vi "CRYGraph Window Menu.vi"(6 "MenuOption":string="View", 8 "pGraph VI":refnum<vi>, 9 "Flag Cluster":T1, 10 "Type":string="View", 11 "Runtime Menu Ref In":refnum<k9>) -> (3 "Runtime Menu Ref Out":refnum<k9>)   [LabVIEW 2013]
uses:
  Control/CRYFlag Cluster.ctl
  System.Windows.Forms
  CRYMainGlobal.vi
  CRYSystem/Task Sequence/CRYProject Run Control Global.vi
panel:
  in  "TextGraph":refnum<k24>(container)
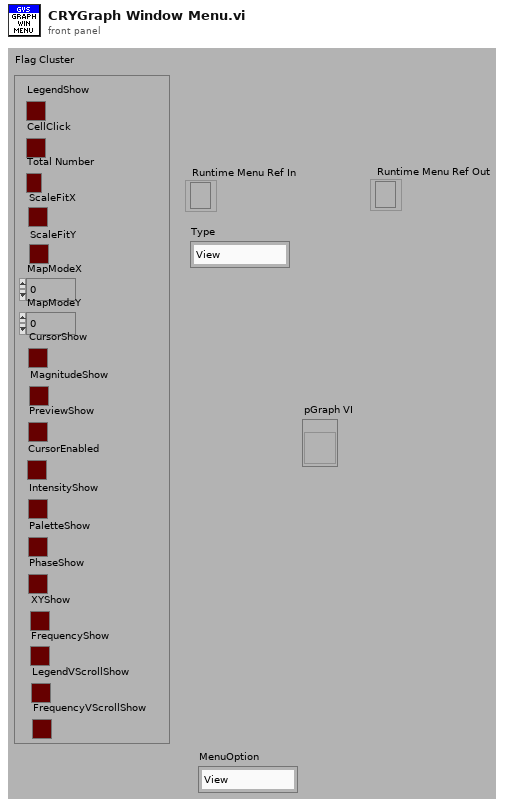
[diagram p1: front panel]
types:
  T1 = typedef "CRYFlag Cluster.ctl" = cluster{"LegendShow":bool, "CellClick":bool, "Total Number":bool, "ScaleFitX":bool, "ScaleFitY":bool, "MapModeX":u8, "MapModeY":u8, "CursorShow":bool, "MagnitudeShow":bool, "PreviewShow":bool, "CursorEnabled":bool, "IntensityShow":bool, "PaletteShow":bool, "PhaseShow":bool, "XYShow":bool, "FrequencyShow":bool, "LegendVScrollShow":bool, "FrequencyVScrollShow":bool}
  T2 = enum32{"English", "Chinese", "Korean", "Japanese", "Russian", "Chinese traditional"}
  T3 = typedef "LVRowAndColumnTypeDef.ctl" = cluster{"Row":i32, "Column":i32}
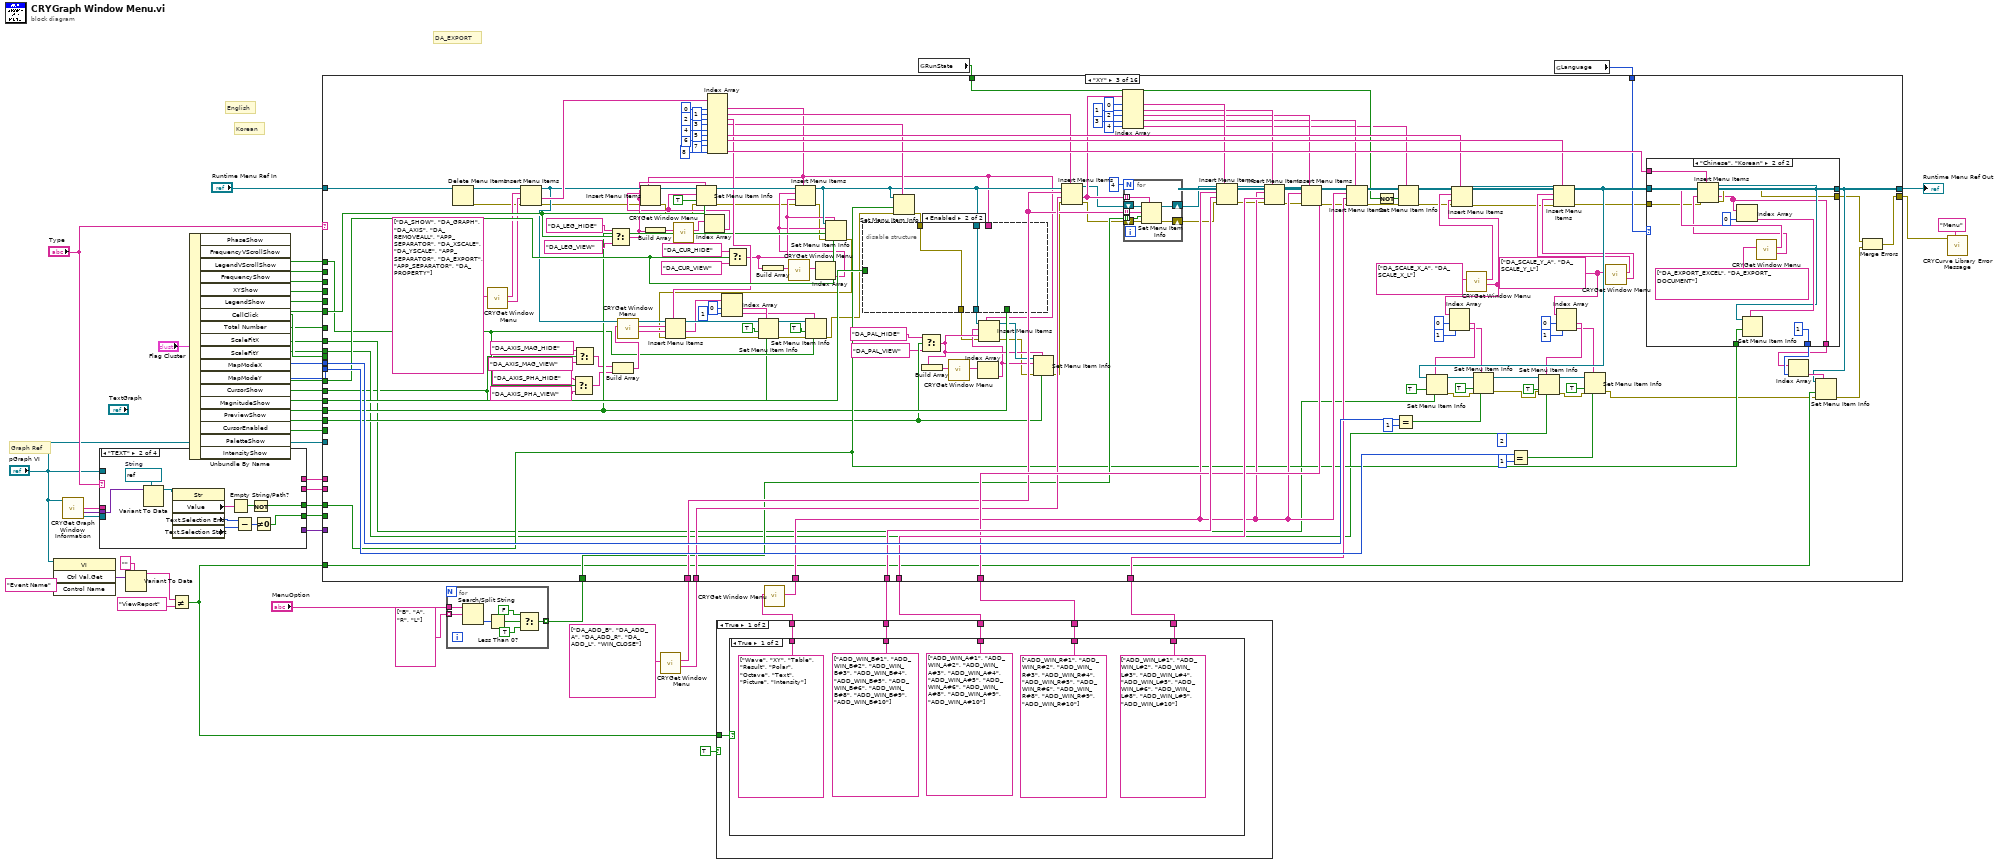
[diagram p0: block diagram]
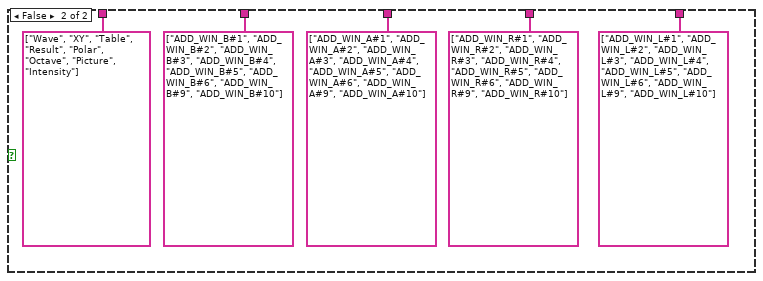
[diagram p2: hidden frame]
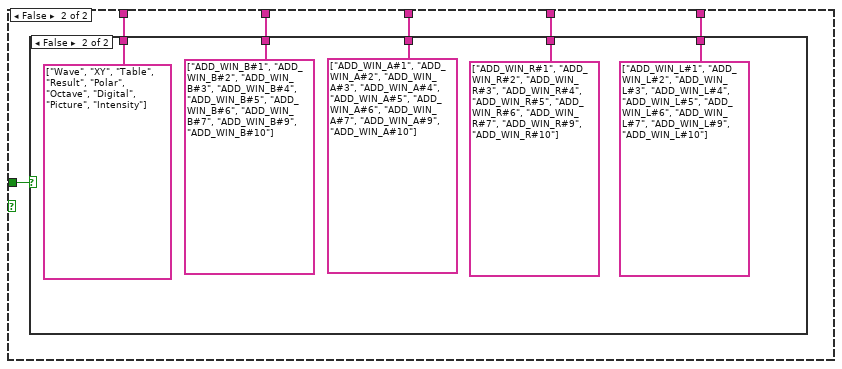
[diagram p3: hidden frame]
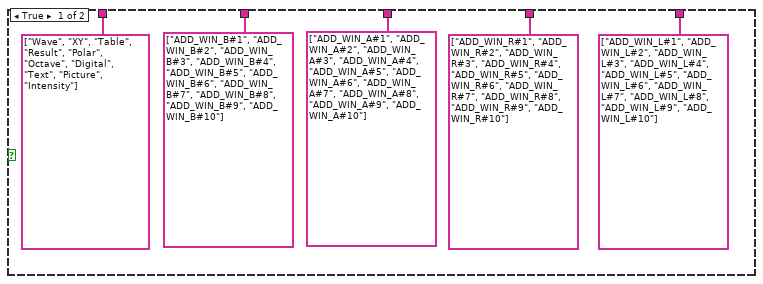
[diagram p4: hidden frame]
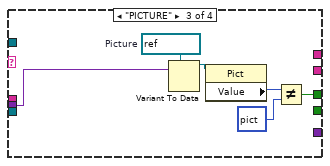
[diagram p6: hidden frame]
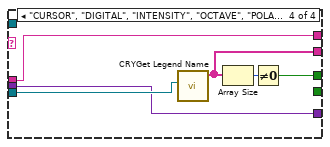
[diagram p7: hidden frame]
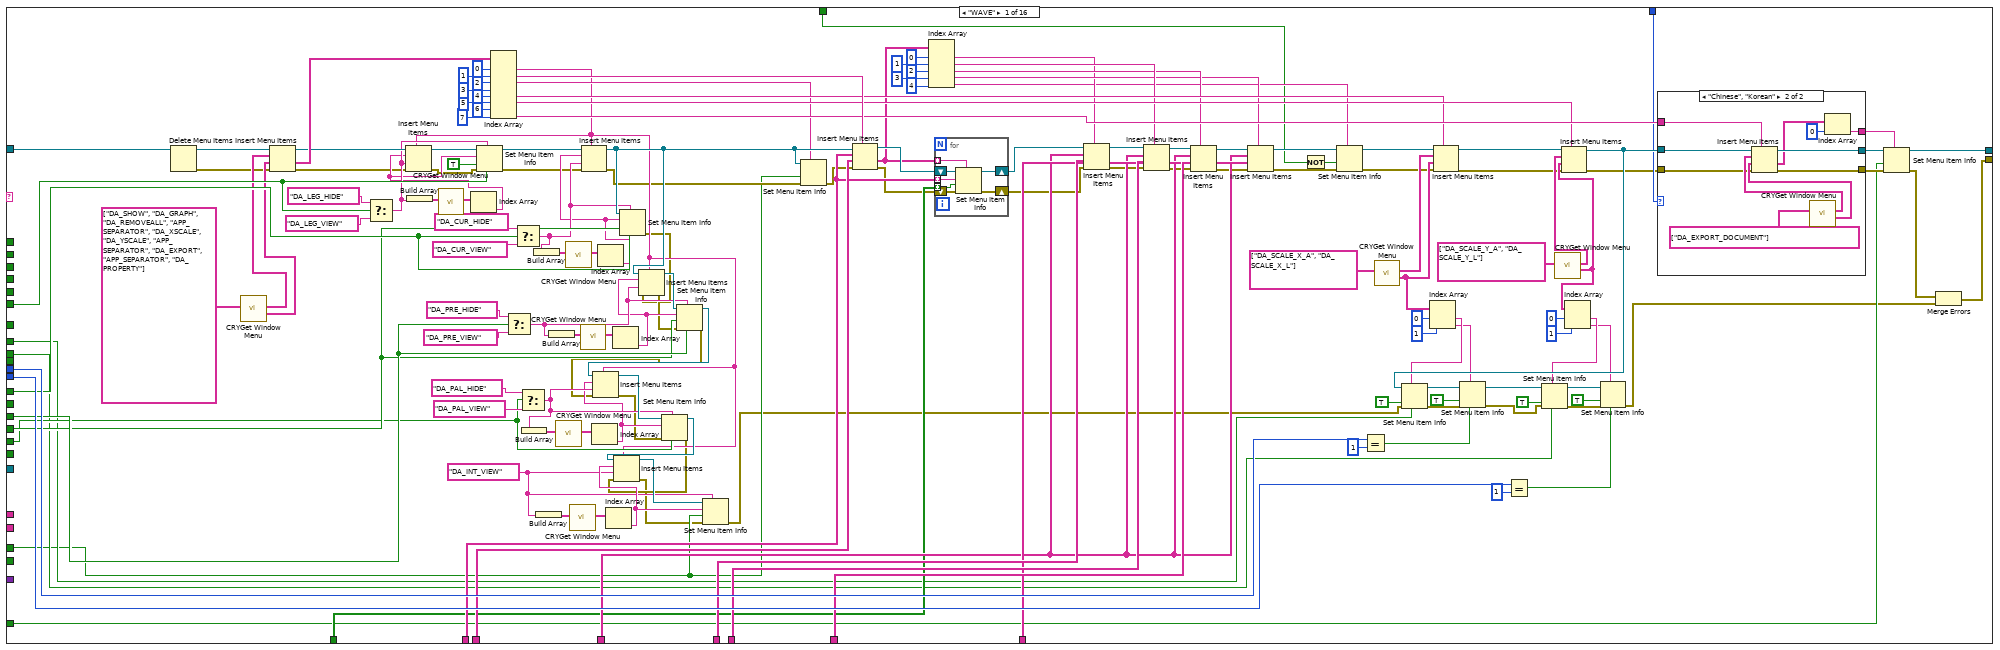
[diagram p8: hidden frame]
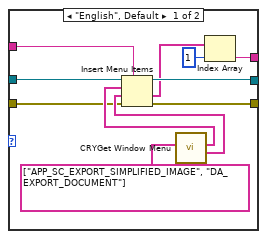
[diagram p9: hidden frame]
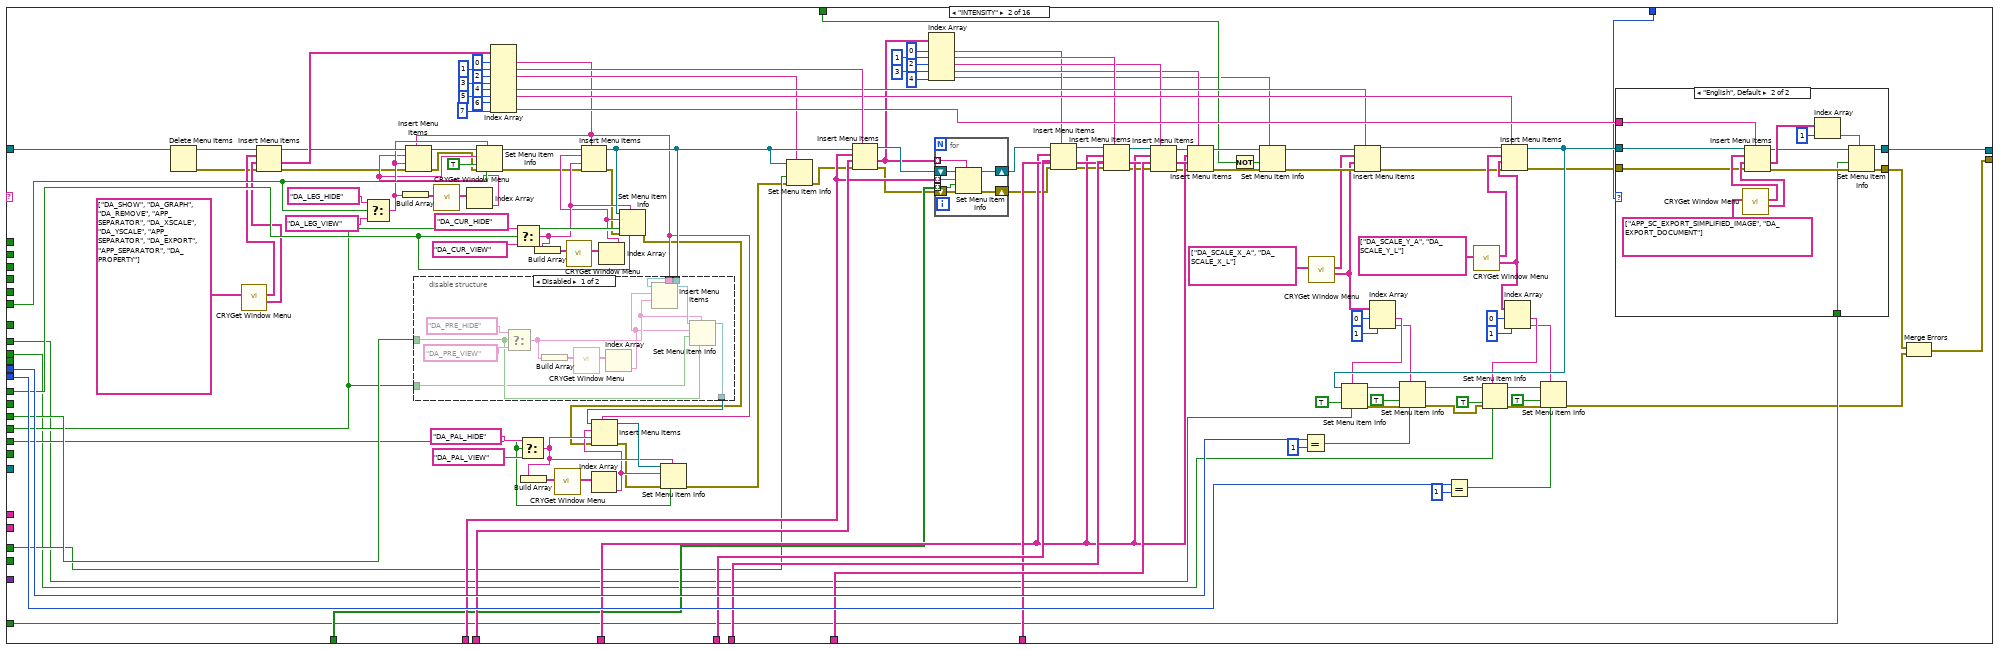
[diagram p10: hidden frame]
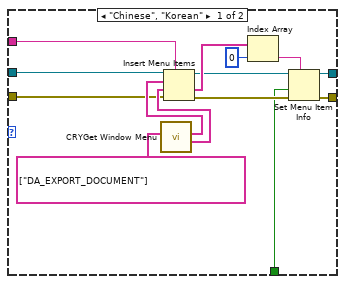
[diagram p11: hidden frame]
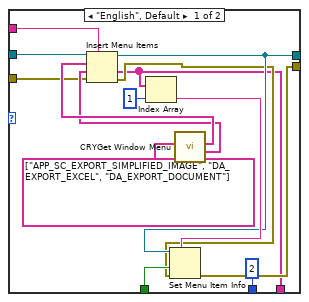
[diagram p13: hidden frame]
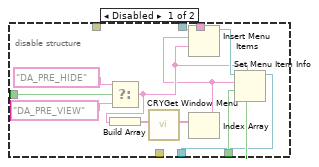
[diagram p14: hidden frame]
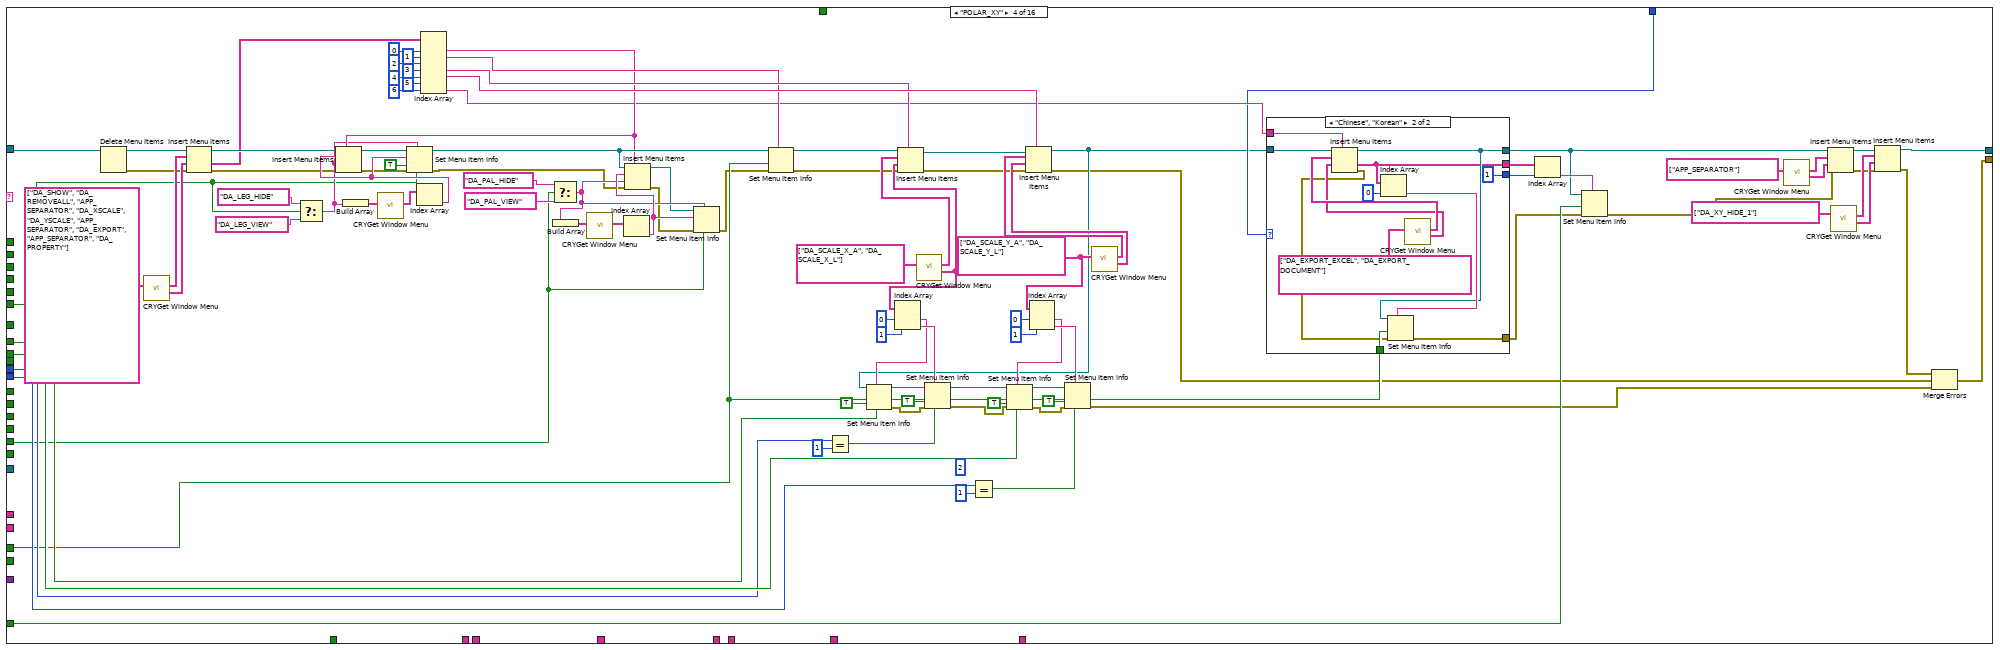
[diagram p15: hidden frame]
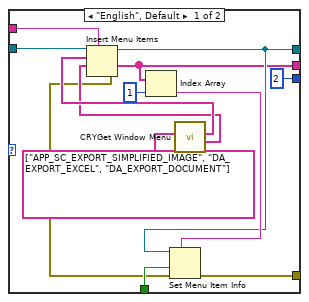
[diagram p16: hidden frame]
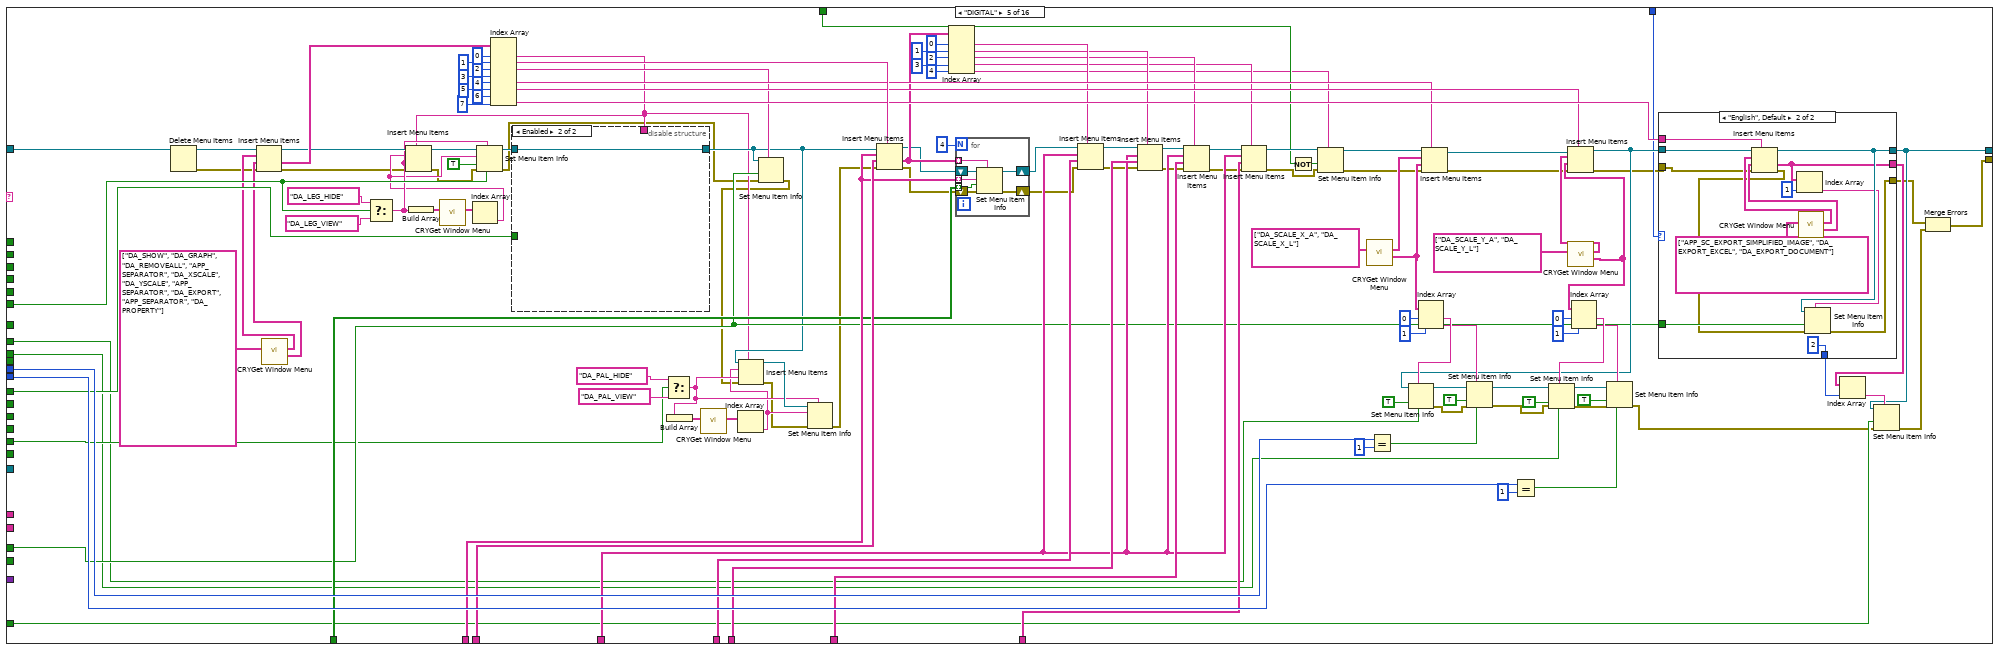
[diagram p17: hidden frame]
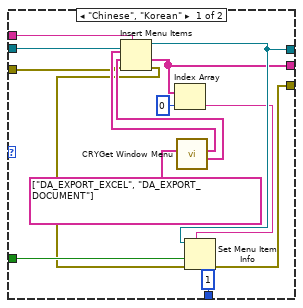
[diagram p18: hidden frame]
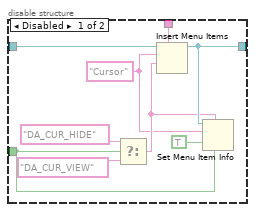
[diagram p19: hidden frame]
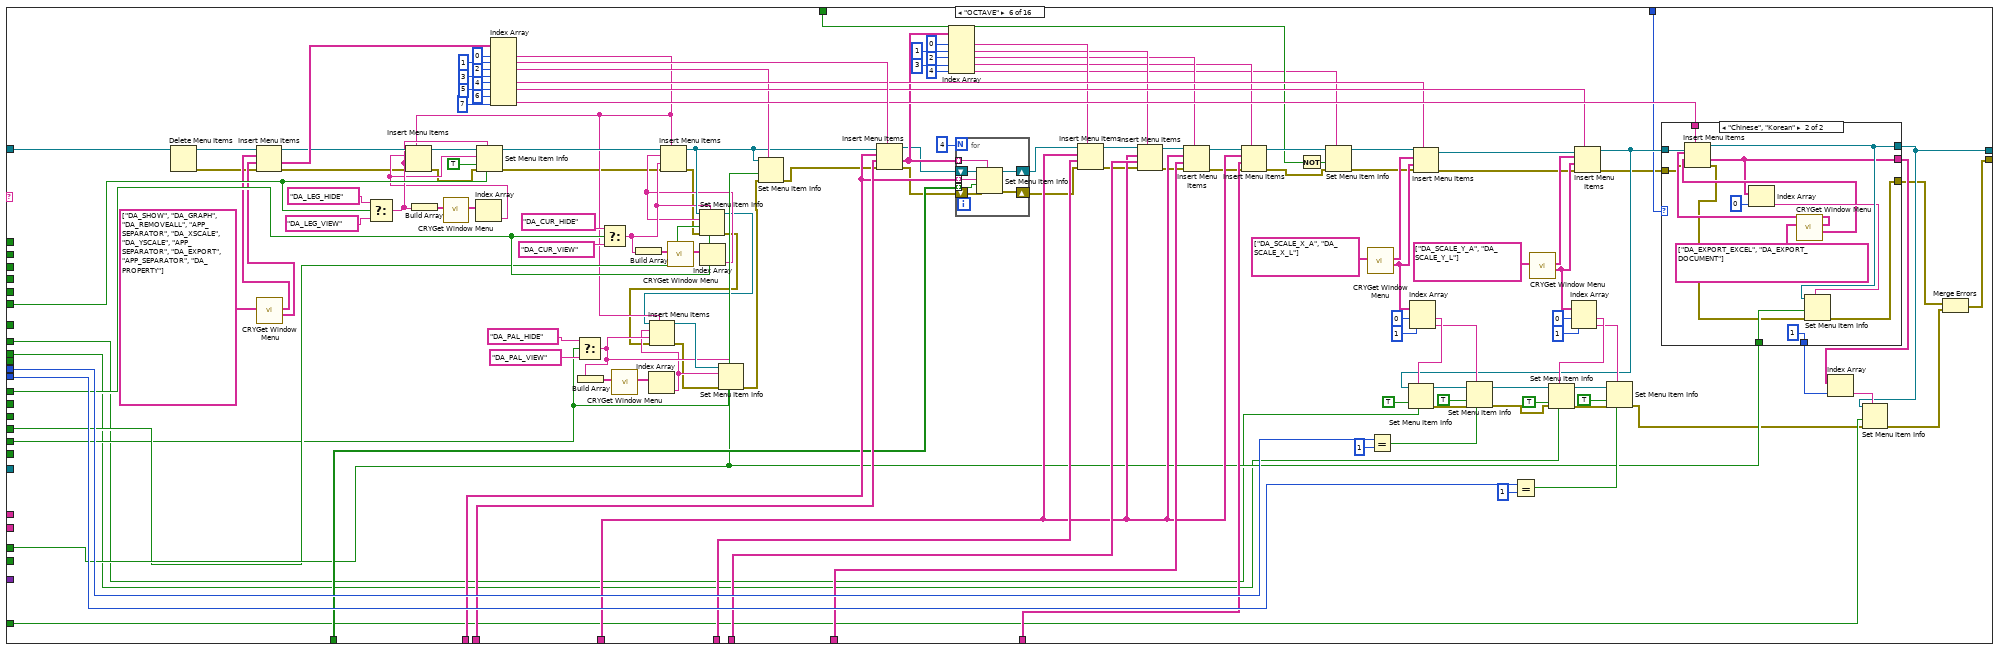
[diagram p20: hidden frame]
diagram:
  # "DA_EXPORT"
  # "Korean"
  # "English"
  # "Graph Ref"
  n1 = invoke class="VI" method="Ctrl Val.Get"(reference="pGraph VI", "Control Name"="Event Name") -> ("Get Control Value Variant"=w11:variant)  [unwired: 2 in, 3 out]
  n2 = call "CRYGet Graph Window Information.vi"("pGraph VI In"="pGraph VI") -> ("Graph Type Out"=w23:string, "Graph Control Ref Out"=w22:variant, "Legend Ref Out"=w21:refnum<vi>)  [unwired: 4 in, 8 out]
  n3 = case shown="\"TEXT\"" "Type" {
    tunnel: "pGraph VI" -> [_ _ _ _]
    tunnel: [_ w58 w67 w76] -> w35
    tunnel: [_ _ _ w75] -> w34
    tunnel: [w55 _ _ w74] -> w33
    tunnel: [_ _ _ w72] -> w32
    tunnel: [_ w57 _ _] -> w30
    tunnel: w23 -> [w55 _ _ w74]
    tunnel: w22 -> [_ w56 w66 w72]
    tunnel: w21 -> [_ _ _ w73]
    frame "INTENSITY_FLOAT", "LEGEND", Default {
    }
    frame "TEXT" {
      w59 = refnum<vi> refnum  # String
      n4 = Variant To Data(type=w59, Variant=w56) -> (data=w60:refnum<vi>)  [unwired: 1 in, 1 out]
      n5 = property class="Str"(reference=w60) -> ("Value"=w65:string, "Text.Selection End"=w61:u32, "Text.Selection Start"=w62:u32)  [unwired: 1 in, 2 out]
      n6 = Empty String/Path?(string/path=w65) -> (empty?=w64:bool)
      n7 = Subtract(x=w61, y=w62) -> (x-y=w63:u32)
      n8 = Not(x=w64) -> (.not. x?=w58:bool)
      n9 = Not Equal To 0?(x=w63) -> (x != 0?=w57:bool)
    }
    frame "PICTURE" {
      w71 = refnum<vi> refnum  # Picture
      n10 = Variant To Data(type=w71, Variant=w66) -> (data=w70:refnum<vi>)  [unwired: 1 in, 1 out]
      n11 = property class="Pict"(reference=w70) -> ("Value"=w69:picture)  [unwired: 1 in, 2 out]
      n12 = Not Equal?(x=w69, y=picture data[5B] ("Value")) -> (x != y?=w67:bool)
    }
    frame "CURSOR", "DIGITAL", "INTENSITY", "OCTAVE", "POLAR", "POLAR_XY", "PREVIEW", "RESULT", "TABLE", "WAVE", "XY" {
      n13 = call "CRYGet Legend Name.vi"("MCListbox Refnum"=w73) -> ("Names Out"=w75:string[])  [unwired: 10 in]
      n14 = Array Size(array=w75) -> (size(s)=w77:i32)
      n15 = Not Equal To 0?(x=w77) -> (x != 0?=w76:bool)
    }
  }
  n16 = Variant To Data(type="" ("Control Name"), Variant=w11) -> (data=w10:string)  [unwired: 1 in, 1 out]
  n17 = Not Equal?(x=w10, y="ViewReport" ("regular expression")) -> (x != y?=w6:bool)
  n18 = Unbundle By Name("Flag Cluster") -> ("PhaseShow"=w4:bool, "FrequencyVScrollShow"=w7:bool, "LegendVScrollShow"=w8:bool, "FrequencyShow"=w16:bool, "XYShow"=w17:bool, "LegendShow"=w52:bool, "CellClick"=w42:bool, "Total Number"=w43:bool, "ScaleFitX"=w19:bool, "ScaleFitY"=w20:bool, "MapModeX"=w50:u8, "MapModeY"=w49:u8, "CursorShow"=w44:bool, "MagnitudeShow"=w41:bool, "PreviewShow"=w40:bool, "CursorEnabled"=w39:bool, "PaletteShow"=w25:bool, "IntensityShow"=w24:bool)
  n19 = for {
    tunnel: "MenuOption" -> [w84]
    tunnel: string[] ["B", "A", "R", "L"] -> [w83] mode=indexing
    tunnel: [w78] -> w37 mode=indexing
    n20 = Search/Split String(string=w84, search string/char (-)=w83) -> (offset of match=w82:i32)  [unwired: 1 in, 2 out]
    n21 = Less Than 0?(x=w82) -> (x < 0?=w81:bool)
    n22 = Select(t=FALSE ("enabled"), s=w81, f=TRUE ("enabled")) -> (s? t:f=w78:bool)
  }
  n23 = call "CRYGet Window Menu.vi"("Tags"=string[] ["DA_ADD_B", "DA_ADD_A", "DA_ADD_R", "DA_ADD_L", "WIN_CLOSE"]) -> ("Tags_Out"=w27:string[], "Names_Out"=w28:string[])  [unwired: 8 in, 1 out]
  n24 = case shown="True" TRUE {
    tunnel: [w90 w106] -> w48
    tunnel: [w89 w105] -> w47
    tunnel: [w88 w104] -> w46
    tunnel: [w87 w103] -> w45
    tunnel: w6 -> [w86 w102]
    tunnel: [w85 w101] -> w5
    frame True {
      n25 = case shown="True" w86 {
        tunnel: [string[] ["ADD_WIN_L#1", "ADD_WIN_L#2", "ADD_WIN_L#3", "ADD_WIN_L#4", "ADD_WIN_L#5", "ADD_WIN_L#6", "ADD_WIN_L#8", "ADD_WIN_L#9", "ADD_WIN_L#10"] string[] ["ADD_WIN_L#1", "ADD_WIN_L#2", "ADD_WIN_L#3", "ADD_WIN_L#4", "ADD_WIN_L#5", "ADD_WIN_L#6", "ADD_WIN_L#9", "ADD_WIN_L#10"]] -> w90
        tunnel: [string[] ["ADD_WIN_R#1", "ADD_WIN_R#2", "ADD_WIN_R#3", "ADD_WIN_R#4", "ADD_WIN_R#5", "ADD_WIN_R#6", "ADD_WIN_R#8", "ADD_WIN_R#9", "ADD_WIN_R#10"] string[] ["ADD_WIN_R#1", "ADD_WIN_R#2", "ADD_WIN_R#3", "ADD_WIN_R#4", "ADD_WIN_R#5", "ADD_WIN_R#6", "ADD_WIN_R#9", "ADD_WIN_R#10"]] -> w89
        tunnel: [string[] ["ADD_WIN_B#1", "ADD_WIN_B#2", "ADD_WIN_B#3", "ADD_WIN_B#4", "ADD_WIN_B#5", "ADD_WIN_B#6", "ADD_WIN_B#8", "ADD_WIN_B#9", "ADD_WIN_B#10"] string[] ["ADD_WIN_B#1", "ADD_WIN_B#2", "ADD_WIN_B#3", "ADD_WIN_B#4", "ADD_WIN_B#5", "ADD_WIN_B#6", "ADD_WIN_B#9", "ADD_WIN_B#10"]] -> w88
        tunnel: [string[] ["ADD_WIN_A#1", "ADD_WIN_A#2", "ADD_WIN_A#3", "ADD_WIN_A#4", "ADD_WIN_A#5", "ADD_WIN_A#6", "ADD_WIN_A#8", "ADD_WIN_A#9", "ADD_WIN_A#10"] string[] ["ADD_WIN_A#1", "ADD_WIN_A#2", "ADD_WIN_A#3", "ADD_WIN_A#4", "ADD_WIN_A#5", "ADD_WIN_A#6", "ADD_WIN_A#9", "ADD_WIN_A#10"]] -> w87
        tunnel: [string[] ["Wave", "XY", "Table", "Result", "Polar", "Octave", "Text", "Picture", "Intensity"] string[] ["Wave", "XY", "Table", "Result", "Polar", "Octave", "Picture", "Intensity"]] -> w85
        frame True {
        }
        frame False {
        }
      }
    }
    frame False {
      n26 = case shown="False" w102 {
        tunnel: [string[] ["ADD_WIN_L#1", "ADD_WIN_L#2", "ADD_WIN_L#3", "ADD_WIN_L#4", "ADD_WIN_L#5", "ADD_WIN_L#6", "ADD_WIN_L#7", "ADD_WIN_L#8", "ADD_WIN_L#9", "ADD_WIN_L#10"] string[] ["ADD_WIN_L#1", "ADD_WIN_L#2", "ADD_WIN_L#3", "ADD_WIN_L#4", "ADD_WIN_L#5", "ADD_WIN_L#6", "ADD_WIN_L#7", "ADD_WIN_L#9", "ADD_WIN_L#10"]] -> w106
        tunnel: [string[] ["ADD_WIN_R#1", "ADD_WIN_R#2", "ADD_WIN_R#3", "ADD_WIN_R#4", "ADD_WIN_R#5", "ADD_WIN_R#6", "ADD_WIN_R#7", "ADD_WIN_R#8", "ADD_WIN_R#9", "ADD_WIN_R#10"] string[] ["ADD_WIN_R#1", "ADD_WIN_R#2", "ADD_WIN_R#3", "ADD_WIN_R#4", "ADD_WIN_R#5", "ADD_WIN_R#6", "ADD_WIN_R#7", "ADD_WIN_R#9", "ADD_WIN_R#10"]] -> w105
        tunnel: [string[] ["ADD_WIN_B#1", "ADD_WIN_B#2", "ADD_WIN_B#3", "ADD_WIN_B#4", "ADD_WIN_B#5", "ADD_WIN_B#6", "ADD_WIN_B#7", "ADD_WIN_B#8", "ADD_WIN_B#9", "ADD_WIN_B#10"] string[] ["ADD_WIN_B#1", "ADD_WIN_B#2", "ADD_WIN_B#3", "ADD_WIN_B#4", "ADD_WIN_B#5", "ADD_WIN_B#6", "ADD_WIN_B#7", "ADD_WIN_B#9", "ADD_WIN_B#10"]] -> w104
        tunnel: [string[] ["ADD_WIN_A#1", "ADD_WIN_A#2", "ADD_WIN_A#3", "ADD_WIN_A#4", "ADD_WIN_A#5", "ADD_WIN_A#6", "ADD_WIN_A#7", "ADD_WIN_A#8", "ADD_WIN_A#9", "ADD_WIN_A#10"] string[] ["ADD_WIN_A#1", "ADD_WIN_A#2", "ADD_WIN_A#3", "ADD_WIN_A#4", "ADD_WIN_A#5", "ADD_WIN_A#6", "ADD_WIN_A#7", "ADD_WIN_A#9", "ADD_WIN_A#10"]] -> w103
        tunnel: [string[] ["Wave", "XY", "Table", "Result", "Polar", "Octave", "Digital", "Text", "Picture", "Intensity"] string[] ["Wave", "XY", "Table", "Result", "Polar", "Octave", "Digital", "Picture", "Intensity"]] -> w101
        frame True {
        }
        frame False {
        }
      }
    }
  }
  n27 = call "CRYGet Window Menu.vi"("Tags"=w5) -> ("Names_Out"=w26:string[])  [unwired: 8 in, 2 out]
  n28 = global read "CRYProject Run Control Global.vi" "RunState"() -> (w15:bool)
  n29 = global read "CRYMainGlobal.vi" "Language"() -> (w18:T2)
  n30 = case shown="\"XY\"" "Type" {
    tunnel: "Runtime Menu Ref In" -> [w269 w435 w644 w736 w950 w1136 w1273 w1372 w1457 w1527 w1600 w1619 w1701 w1737 w1832 w1835]
    tunnel: w52 -> [w222 w409 w596 w735 w902 w1088 _ _ _ _ _ _ _ _ _ _]
    tunnel: w43 -> [_ _ _ _ _ _ _ _ _ _ _ w1615 w1698 _ _ _]
    tunnel: [w133 w309 w509 w729 w838 w1014 w1184 w1294 w1384 w1469 w1537 w1620 w1702 w1735 w1830 w1834] -> w53
    tunnel: w50 -> [w242 w427 w617 w732 w923 w1109 _ _ _ _ _ _ _ _ _ _]
    tunnel: w49 -> [w240 w426 w615 w731 w921 w1107 _ _ _ _ _ _ _ _ _ _]
    tunnel: w42 -> [_ _ _ _ _ _ _ _ _ _ _ w1616 w1699 _ _ _]
    tunnel: w19 -> [w166 w371 w543 w734 w866 w1044 _ _ _ _ _ _ _ _ _ _]
    tunnel: w20 -> [w165 w370 w542 w733 w865 w1043 _ _ _ _ _ _ _ _ _ _]
    tunnel: w48 -> [w225 w412 w599 _ w905 w1091 w1255 w1364 w1449 w1520 w1594 _ _ _ _ _]
    tunnel: w47 -> [w226 w413 w600 _ w906 w1092 w1256 w1363 w1448 w1519 w1593 _ _ _ _ _]
    tunnel: w46 -> [w228 w415 w602 _ w908 w1094 w1258 w1362 w1447 w1518 w1592 _ _ _ _ _]
    tunnel: w45 -> [w227 w414 w601 _ w907 w1093 w1257 w1361 w1446 w1517 w1591 _ _ _ _ _]
    tunnel: w28 -> [w209 w399 w579 _ w896 w1082 w1246 w1347 w1432 w1504 w1578 _ _ _ _ _]
    tunnel: w27 -> [w223 w410 w597 _ w903 w1089 w1253 w1360 w1445 w1516 w1590 _ _ _ _ _]
    tunnel: w26 -> [w224 w411 w598 _ w904 w1090 w1254 w1359 w1444 w1515 w1589 _ _ _ _ _]
    tunnel: w44 -> [w217 w404 w591 _ w899 w1085 _ _ _ _ _ _ _ w1734 _ _]
    tunnel: w41 -> [_ _ w492 _ _ _ _ _ _ _ _ _ _ _ _ _]
    tunnel: w40 -> [w213 w403 w576 _ _ _ _ _ _ _ _ _ _ _ _ _]
    tunnel: w39 -> [w206 w396 w574 _ _ w1072 _ _ _ _ _ _ _ _ _ _]
    tunnel: w37 -> [w208 w398 w578 _ w895 w1081 w1245 w1346 w1431 w1503 w1577 _ _ _ _ _]
    tunnel: w35 -> [w149 w393 w575 w726 w890 w1075 w1189 w1298 w1414 w1499 w1567 _ _ _ _ _]
    tunnel: w34 -> [_ _ _ _ _ _ _ _ _ _ _ _ _ w1730 _ _]
    tunnel: w33 -> [_ _ _ _ _ _ _ _ _ _ _ w1609 w1697 w1725 _ _]
    tunnel: w32 -> [_ _ _ _ _ _ _ w1328 _ _ _ _ _ w1729 _ _]
    tunnel: w30 -> [_ _ _ _ _ _ _ _ _ _ w1566 _ _ _ _ _]
    tunnel: w25 -> [w175 w372 w546 w730 w867 w1047 _ _ _ _ _ _ _ _ _ _]
    tunnel: w24 -> [_ _ _ _ _ _ _ _ _ _ _ _ _ _ _ _]
    tunnel: "pGraph VI" -> [_ _ _ _ _ _ _ _ w1418 _ _ _ _ _ _ _]
    tunnel: w18 -> [w164 w307 w541 w727 w864 w1042 _ _ _ _ _ _ _ _ _ _]
    tunnel: [w117 w302 w489 w702 w830 w1006 w1183 w1292 w1382 w1467 w1536 w1611 w1676 w1721 w1825 w1833] -> w2
    tunnel: w17 -> [_ _ _ _ _ _ w1215 _ _ _ _ _ _ _ _ _]
    tunnel: w16 -> [_ _ _ _ _ _ w1214 _ _ _ _ _ _ _ _ _]
    tunnel: w15 -> [w144 w349 w515 _ w842 w1020 w1200 w1307 w1397 w1484 w1543 _ _ _ _ _]
    tunnel: w6 -> [w130 w308 w508 w720 w835 w1011 w1182 w1291 w1381 w1466 _ _ _ _ _ _]
    tunnel: w8 -> [_ _ _ _ _ _ _ _ _ _ _ w1610 _ _ _ _]
    tunnel: w7 -> [_ _ _ _ _ _ _ _ _ _ _ _ w1675 _ _ _]
    tunnel: w4 -> [_ _ w493 _ _ _ _ _ _ _ _ _ _ _ _ _]
    frame "WAVE" {
      w167 = "DA_INT_VIEW"
      n31 = Delete Menu Items(9:w269) -> (0:w163:errorcluster, 3:w272:refnum<k9>)  [unwired: 1 in, 2 out]
      n32 = call "CRYGet Window Menu.vi"("Tags"=string[] ["DA_SHOW", "DA_GRAPH", "DA_REMOVEALL", "APP_SEPARATOR", "DA_XSCALE", "DA_YSCALE", "APP_SEPARATOR", "DA_EXPORT", "APP_SEPARATOR", "DA_PROPERTY"]) -> ("Tags_Out"=w201:string[], "Names_Out"=w202:string[])  [unwired: 8 in, 1 out]
      n33 = Insert Menu Items(6:w163, 7:w201, 8:w202, 9:w272) -> (0:w162:errorcluster, 1:w271:string[], 3:w268:refnum<k9>)  [unwired: 2 out]
      n34 = Select(t="DA_LEG_HIDE", s=w222, f="DA_LEG_VIEW") -> (s? t:f=w198:string)
      n35 = Build Array(w198) -> (w200:string[])
      n36 = call "CRYGet Window Menu.vi"("Tags"=w200) -> ("Names_Out"=w199:string[])  [unwired: 8 in, 2 out]
      n37 = Index Array(array=w199) -> (element=w197:string)  [unwired: 1 in]
      n38 = Index Array(array=w271, index #1=0 ("index"), index #2=1 ("index"), index #3=2 ("index"), index #4=3 ("index"), index #5=4 ("index"), index #6=5 ("index"), index #7=6 ("index"), index #8=7 ("index")) -> (element #1=w169:string, element #2=w270:string, element #3=w204:string, element #5=w253:string, element #6=w254:string, element #8=w264:string)  [unwired: 2 out]
      n39 = Insert Menu Items(5:w169, 6:w162, 7:w198, 8:w197, 9:w268) -> (0:w161:errorcluster, 3:w267:refnum<k9>)  [unwired: 1 in, 1 out]
      n40 = Set Menu Item Info(6:w222, 7:w198, 8:w161, 9:TRUE ("enabled"), 10:w197, 11:w267) -> (0:w160:errorcluster, 3:w266:refnum<k9>)  [unwired: 1 out]
      n41 = Select(t="DA_PRE_HIDE", s=w213, f="DA_PRE_VIEW") -> (s? t:f=w184:string)
      n42 = Select(t="DA_CUR_HIDE", s=w217, f="DA_CUR_VIEW") -> (s? t:f=w194:string)
      n43 = Select(t="DA_PAL_HIDE", s=w175, f="DA_PAL_VIEW") -> (s? t:f=w179:string)
      n44 = Build Array(w179) -> (w182:string[])
      n45 = Build Array(w194) -> (w196:string[])
      n46 = Build Array(w167) -> (w172:string[])
      n47 = Build Array(w184) -> (w185:string[])
      n48 = call "CRYGet Window Menu.vi"("Tags"=w182) -> ("Names_Out"=w181:string[])  [unwired: 8 in, 2 out]
      n49 = call "CRYGet Window Menu.vi"("Tags"=w196) -> ("Names_Out"=w195:string[])  [unwired: 8 in, 2 out]
      n50 = call "CRYGet Window Menu.vi"("Tags"=w172) -> ("Names_Out"=w173:string[])  [unwired: 8 in, 2 out]
      n51 = call "CRYGet Window Menu.vi"("Tags"=w185) -> ("Names_Out"=w186:string[])  [unwired: 8 in, 2 out]
      n52 = Index Array(array=w181) -> (element=w178:string)  [unwired: 1 in]
      n53 = Index Array(array=w195) -> (element=w193:string)  [unwired: 1 in]
      n54 = Insert Menu Items(5:w169, 6:w160, 7:w194, 8:w193, 9:w266) -> (0:w159:errorcluster, 3:w205:refnum<k9>)  [unwired: 2 out]
      n55 = Index Array(array=w173) -> (element=w168:string)  [unwired: 1 in]
      n56 = Index Array(array=w186) -> (element=w183:string)  [unwired: 1 in]
      n57 = Set Menu Item Info(6:w217, 7:w194, 9:w206, 10:w193, 11:w205) -> (0:w124:errorcluster)  [unwired: 1 in, 2 out]
      n58 = Insert Menu Items(5:w169, 6:w124, 7:w184, 8:w183, 9:w205) -> (0:w129:errorcluster, 3:w214:refnum<k9>)  [unwired: 2 out]
      n59 = Set Menu Item Info(6:w213, 7:w184, 8:w129, 9:w206, 10:w183, 11:w214) -> (0:w128:errorcluster, 3:w174:refnum<k9>)  [unwired: 1 out]
      n60 = Insert Menu Items(5:w169, 6:w128, 7:w179, 8:w178, 9:w174) -> (0:w127:errorcluster, 3:w180:refnum<k9>)  [unwired: 2 out]
      n61 = Set Menu Item Info(6:w175, 7:w179, 8:w127, 10:w178, 11:w180) -> (0:w126:errorcluster, 3:w171:refnum<k9>)  [unwired: 1 in, 1 out]
      n62 = Insert Menu Items(5:w169, 6:w126, 7:w167, 8:w168, 9:w171) -> (0:w125:errorcluster, 3:w170:refnum<k9>)  [unwired: 2 out]
      n63 = Set Menu Item Info(7:w167, 8:w125, 9:w149, 10:w168, 11:w170) -> (0:w123:errorcluster)  [unwired: 1 in, 2 out]
      n64 = Set Menu Item Info(7:w204, 8:w159, 9:w149, 11:w205) -> (0:w158:errorcluster)  [unwired: 1 in, 3 out]
      n65 = Insert Menu Items(5:w270, 6:w158, 7:w223, 8:w209, 9:w205) -> (0:w157:errorcluster, 1:w210:string[], 3:w211:refnum<k9>)  [unwired: 1 out]
      n66 = Index Array(array=w210, index #1=0 ("index"), index #2=1 ("index"), index #3=2 ("index"), index #4=3 ("index"), index #5=4 ("index")) -> (element #1=w212:string, element #2=w234:string, element #3=w233:string, element #4=w232:string, element #5=w145:string)
      n67 = for {
        tunnel: w210 -> [w300] mode=indexing
        tunnel: w209 -> [w299] mode=indexing
        tunnel: w208 -> [w298] mode=indexing
        shift-right: [w297] -> w207
        shift-left: w211 -> [w301]
        shift-right: [w295] -> w156
        shift-left: w157 -> [w296]
        n68 = Set Menu Item Info(7:w300, 8:w296, 9:w298, 10:w299, 11:w301) -> (0:w295:errorcluster, 3:w297:refnum<k9>)  [unwired: 1 in, 1 out]
      }
      n69 = Insert Menu Items(5:w212, 6:w156, 7:w228, 8:w224, 9:w207) -> (0:w155:errorcluster, 3:w231:refnum<k9>)  [unwired: 2 out]
      n70 = Insert Menu Items(5:w234, 6:w155, 7:w227, 8:w224, 9:w231) -> (0:w154:errorcluster, 3:w230:refnum<k9>)  [unwired: 2 out]
      n71 = Insert Menu Items(5:w233, 6:w154, 7:w226, 8:w224, 9:w230) -> (0:w153:errorcluster, 3:w229:refnum<k9>)  [unwired: 2 out]
      n72 = Insert Menu Items(5:w232, 6:w153, 7:w225, 8:w224, 9:w229) -> (0:w152:errorcluster, 3:w147:refnum<k9>)  [unwired: 2 out]
      n73 = Not(x=w144) -> (.not. x?=w143:bool)
      n74 = Set Menu Item Info(7:w145, 9:w143, 11:w147) -> (3:w146:refnum<k9>)  [unwired: 2 in, 3 out]
      n75 = Equal?(x=w242, y=u8 1) -> (x = y?=w241:bool)
      n76 = call "CRYGet Window Menu.vi"("Tags"=string[] ["DA_SCALE_X_A", "DA_SCALE_X_L"]) -> ("Tags_Out"=w190:string[], "Names_Out"=w191:string[])  [unwired: 8 in, 1 out]
      n77 = Index Array(array=w190, index #1=0 ("index"), index #2=1 ("index")) -> (element #1=w250:string, element #2=w249:string)
      n78 = Insert Menu Items(5:w253, 6:w152, 7:w190, 8:w191, 9:w146) -> (0:w151:errorcluster, 3:w263:refnum<k9>)  [unwired: 2 out]
      n79 = Equal?(x=w240, y=u8 1) -> (x = y?=w239:bool)
      n80 = call "CRYGet Window Menu.vi"("Tags"=string[] ["DA_SCALE_Y_A", "DA_SCALE_Y_L"]) -> ("Tags_Out"=w187:string[], "Names_Out"=w188:string[])  [unwired: 8 in, 1 out]
      n81 = Insert Menu Items(5:w254, 6:w151, 7:w187, 8:w188, 9:w263) -> (0:w150:errorcluster, 3:w261:refnum<k9>)  [unwired: 2 out]
      n82 = Set Menu Item Info(6:w166, 7:w250, 8:w123, 9:TRUE ("enabled"), 11:w261) -> (0:w122:errorcluster, 3:w260:refnum<k9>)  [unwired: 2 out]
      n83 = Set Menu Item Info(6:w241, 7:w249, 8:w122, 9:TRUE ("enabled"), 11:w260) -> (0:w121:errorcluster, 3:w256:refnum<k9>)  [unwired: 2 out]
      n84 = Index Array(array=w187, index #1=0 ("index"), index #2=1 ("index")) -> (element #1=w246:string, element #2=w245:string)
      n85 = Set Menu Item Info(6:w165, 7:w246, 8:w121, 9:TRUE ("enabled"), 11:w256) -> (0:w120:errorcluster, 3:w255:refnum<k9>)  [unwired: 2 out]
      n86 = Set Menu Item Info(6:w239, 7:w245, 8:w120, 9:TRUE ("enabled"), 11:w255) -> (0:w118:errorcluster)  [unwired: 3 out]
      n87 = case shown="\"Chinese\", \"Korean\"" w164 {
        tunnel: w264 -> [w283 w294]
        tunnel: w261 -> [w282 w293]
        tunnel: [w281 w292] -> w134
        tunnel: w150 -> [w278 w289]
        tunnel: [w277 w288] -> w132
        tunnel: [w273 w284] -> w131
        frame "English", Default {
          n88 = call "CRYGet Window Menu.vi"("Tags"=string[] ["APP_SC_EXPORT_SIMPLIFIED_IMAGE", "DA_EXPORT_DOCUMENT"]) -> ("Tags_Out"=w279:string[], "Names_Out"=w280:string[])  [unwired: 8 in, 1 out]
          n89 = Insert Menu Items(5:w283, 6:w278, 7:w279, 8:w280, 9:w282) -> (0:w277:errorcluster, 1:w274:string[], 3:w281:refnum<k9>)  [unwired: 1 out]
          n90 = Index Array(array=w274, index=1) -> (element=w273:string)
        }
        frame "Chinese", "Korean" {
          n91 = call "CRYGet Window Menu.vi"("Tags"=string[] ["DA_EXPORT_DOCUMENT"]) -> ("Tags_Out"=w290:string[], "Names_Out"=w291:string[])  [unwired: 8 in, 1 out]
          n92 = Insert Menu Items(5:w294, 6:w289, 7:w290, 8:w291, 9:w293) -> (0:w288:errorcluster, 1:w285:string[], 3:w292:refnum<k9>)  [unwired: 1 out]
          n93 = Index Array(array=w285, index=0) -> (element=w284:string)
        }
      }
      n94 = Set Menu Item Info(7:w131, 8:w132, 9:w130, 11:w134) -> (0:w119:errorcluster, 3:w133:refnum<k9>)  [unwired: 2 in, 1 out]
      n95 = Merge Errors(w119, w118) -> (w117:errorcluster)
    }
    frame "INTENSITY" {
      n96 = Delete Menu Items(9:w435) -> (0:w369:errorcluster, 3:w438:refnum<k9>)  [unwired: 1 in, 2 out]
      n97 = call "CRYGet Window Menu.vi"("Tags"=string[] ["DA_SHOW", "DA_GRAPH", "DA_REMOVE", "APP_SEPARATOR", "DA_XSCALE", "DA_YSCALE", "APP_SEPARATOR", "DA_EXPORT", "APP_SEPARATOR", "DA_PROPERTY"]) -> ("Tags_Out"=w390:string[], "Names_Out"=w391:string[])  [unwired: 8 in, 1 out]
      n98 = Insert Menu Items(6:w369, 7:w390, 8:w391, 9:w438) -> (0:w368:errorcluster, 1:w437:string[], 3:w434:refnum<k9>)  [unwired: 2 out]
      n99 = Select(t="DA_LEG_HIDE", s=w409, f="DA_LEG_VIEW") -> (s? t:f=w387:string)
      n100 = Build Array(w387) -> (w389:string[])
      n101 = call "CRYGet Window Menu.vi"("Tags"=w389) -> ("Names_Out"=w388:string[])  [unwired: 8 in, 2 out]
      n102 = Index Array(array=w388) -> (element=w386:string)  [unwired: 1 in]
      n103 = Index Array(array=w437, index #1=0 ("index"), index #2=1 ("index"), index #3=2 ("index"), index #4=3 ("index"), index #5=4 ("index"), index #6=5 ("index"), index #7=6 ("index"), index #8=7 ("index")) -> (element #1=w374:string, element #2=w436:string, element #3=w394:string, element #5=w428:string, element #6=w429:string, element #8=w430:string)  [unwired: 2 out]
      n104 = Insert Menu Items(5:w374, 6:w368, 7:w387, 8:w386, 9:w434) -> (0:w367:errorcluster, 3:w433:refnum<k9>)  [unwired: 1 in, 1 out]
      n105 = Set Menu Item Info(6:w409, 7:w387, 8:w367, 9:TRUE ("enabled"), 10:w386, 11:w433) -> (0:w366:errorcluster, 3:w432:refnum<k9>)  [unwired: 1 out]
      n106 = Select(t="DA_CUR_HIDE", s=w404, f="DA_CUR_VIEW") -> (s? t:f=w383:string)
      n107 = Select(t="DA_PAL_HIDE", s=w372, f="DA_PAL_VIEW") -> (s? t:f=w378:string)
      n108 = Build Array(w378) -> (w381:string[])
      n109 = Build Array(w383) -> (w385:string[])
      n110 = call "CRYGet Window Menu.vi"("Tags"=w381) -> ("Names_Out"=w380:string[])  [unwired: 8 in, 2 out]
      n111 = call "CRYGet Window Menu.vi"("Tags"=w385) -> ("Names_Out"=w384:string[])  [unwired: 8 in, 2 out]
      n112 = Index Array(array=w380) -> (element=w377:string)  [unwired: 1 in]
      n113 = Index Array(array=w384) -> (element=w382:string)  [unwired: 1 in]
      n114 = Insert Menu Items(5:w374, 6:w366, 7:w383, 8:w382, 9:w432) -> (0:w365:errorcluster, 3:w395:refnum<k9>)  [unwired: 2 out]
      n115 = disable-structure shown="Disabled" {
        disable-tunnel: w403 -> [w475 _]
        disable-tunnel: w396 -> [w474 _]
        disable-tunnel: w395 -> [w473 w479]
        disable-tunnel: w374 -> [w468 _]
        disable-tunnel: [w467 w479] -> w373
        frame Disabled {
          n116 = Select(t="DA_PRE_HIDE", s=w475, f="DA_PRE_VIEW") -> (s? t:f=w470:string)
          n117 = Build Array(w470) -> (w472:string[])
          n118 = call "CRYGet Window Menu.vi"("Tags"=w472) -> ("Names_Out"=w471:string[])  [unwired: 8 in, 2 out]
          n119 = Index Array(array=w471) -> (element=w469:string)  [unwired: 1 in]
          n120 = Insert Menu Items(5:w468, 7:w470, 8:w469, 9:w473) -> (3:w476:refnum<k9>)  [unwired: 1 in, 3 out]
          n121 = Set Menu Item Info(6:w475, 7:w470, 9:w474, 10:w469, 11:w476) -> (3:w467:refnum<k9>)  [unwired: 1 in, 2 out]
        }
        frame Enabled {
        }
      }
      n122 = Set Menu Item Info(6:w404, 7:w383, 8:w365, 9:w396, 10:w382, 11:w395) -> (0:w358:errorcluster)  [unwired: 2 out]
      n123 = Insert Menu Items(5:w374, 6:w358, 7:w378, 8:w377, 9:w373) -> (0:w357:errorcluster, 3:w379:refnum<k9>)  [unwired: 2 out]
      n124 = Set Menu Item Info(6:w372, 7:w378, 8:w357, 10:w377, 11:w379) -> (0:w356:errorcluster)  [unwired: 1 in, 2 out]
      n125 = Set Menu Item Info(7:w394, 8:w356, 9:w393, 11:w395) -> (0:w364:errorcluster)  [unwired: 1 in, 3 out]
      n126 = Insert Menu Items(5:w436, 6:w364, 7:w410, 8:w399, 9:w395) -> (0:w363:errorcluster, 1:w400:string[], 3:w401:refnum<k9>)  [unwired: 1 out]
      n127 = Index Array(array=w400, index #1=0 ("index"), index #2=1 ("index"), index #3=2 ("index"), index #4=3 ("index"), index #5=4 ("index")) -> (element #1=w402:string, element #2=w421:string, element #3=w420:string, element #4=w419:string, element #5=w348:string)
      n128 = for {
        tunnel: w400 -> [w485] mode=indexing
        tunnel: w399 -> [w484] mode=indexing
        tunnel: w398 -> [w483] mode=indexing
        shift-right: [w482] -> w397
        shift-left: w401 -> [w486]
        shift-right: [w480] -> w362
        shift-left: w363 -> [w481]
        n129 = Set Menu Item Info(7:w485, 8:w481, 9:w483, 10:w484, 11:w486) -> (0:w480:errorcluster, 3:w482:refnum<k9>)  [unwired: 1 in, 1 out]
      }
      n130 = Insert Menu Items(5:w402, 6:w362, 7:w415, 8:w411, 9:w397) -> (0:w361:errorcluster, 3:w418:refnum<k9>)  [unwired: 2 out]
      n131 = Insert Menu Items(5:w421, 6:w361, 7:w414, 8:w411, 9:w418) -> (0:w360:errorcluster, 3:w417:refnum<k9>)  [unwired: 2 out]
      n132 = Insert Menu Items(5:w420, 6:w360, 7:w413, 8:w411, 9:w417) -> (0:w359:errorcluster, 3:w416:refnum<k9>)  [unwired: 2 out]
      n133 = Insert Menu Items(5:w419, 6:w359, 7:w412, 8:w411, 9:w416) -> (0:w351:errorcluster, 3:w353:refnum<k9>)  [unwired: 2 out]
      n134 = Not(x=w349) -> (.not. x?=w354:bool)
      n135 = Set Menu Item Info(7:w348, 8:w351, 9:w354, 11:w353) -> (0:w350:errorcluster, 3:w352:refnum<k9>)  [unwired: 1 in, 2 out]
      n136 = Equal?(x=w427, y=u8 1) -> (x = y?=w320:bool)
      n137 = call "CRYGet Window Menu.vi"("Tags"=string[] ["DA_SCALE_X_A", "DA_SCALE_X_L"]) -> ("Tags_Out"=w316:string[], "Names_Out"=w317:string[])  [unwired: 8 in, 1 out]
      n138 = Insert Menu Items(5:w428, 6:w350, 7:w316, 8:w317, 9:w352) -> (0:w306:errorcluster, 3:w339:refnum<k9>)  [unwired: 2 out]
      n139 = Index Array(array=w316, index #1=0 ("index"), index #2=1 ("index")) -> (element #1=w328:string, element #2=w327:string)
      n140 = Equal?(x=w426, y=u8 1) -> (x = y?=w319:bool)
      n141 = call "CRYGet Window Menu.vi"("Tags"=string[] ["DA_SCALE_Y_A", "DA_SCALE_Y_L"]) -> ("Tags_Out"=w313:string[], "Names_Out"=w314:string[])  [unwired: 8 in, 1 out]
      n142 = Insert Menu Items(5:w429, 6:w306, 7:w313, 8:w314, 9:w339) -> (0:w305:errorcluster, 3:w337:refnum<k9>)  [unwired: 2 out]
      n143 = Set Menu Item Info(6:w371, 7:w328, 9:TRUE ("enabled"), 11:w337) -> (0:w312:errorcluster, 3:w336:refnum<k9>)  [unwired: 1 in, 2 out]
      n144 = Set Menu Item Info(6:w320, 7:w327, 8:w312, 9:TRUE ("enabled"), 11:w336) -> (0:w311:errorcluster, 3:w332:refnum<k9>)  [unwired: 2 out]
      n145 = Index Array(array=w313, index #1=0 ("index"), index #2=1 ("index")) -> (element #1=w324:string, element #2=w323:string)
      n146 = Set Menu Item Info(6:w370, 7:w324, 8:w311, 9:TRUE ("enabled"), 11:w332) -> (0:w310:errorcluster, 3:w331:refnum<k9>)  [unwired: 2 out]
      n147 = Set Menu Item Info(6:w319, 7:w323, 8:w310, 9:TRUE ("enabled"), 11:w331) -> (0:w303:errorcluster)  [unwired: 3 out]
      n148 = case shown="\"English\", Default" w307 {
        tunnel: w430 -> [w452 w466]
        tunnel: w337 -> [w451 w465]
        tunnel: w305 -> [w447 w461]
        tunnel: [w442 w456] -> w309
        tunnel: [w440 w454] -> w304
        tunnel: w308 -> [w439 w453]
        frame "Chinese", "Korean" {
          n149 = call "CRYGet Window Menu.vi"("Tags"=string[] ["DA_EXPORT_DOCUMENT"]) -> ("Tags_Out"=w448:string[], "Names_Out"=w449:string[])  [unwired: 8 in, 1 out]
          n150 = Insert Menu Items(5:w452, 6:w447, 7:w448, 8:w449, 9:w451) -> (0:w441:errorcluster, 1:w445:string[], 3:w443:refnum<k9>)  [unwired: 1 out]
          n151 = Index Array(array=w445, index=0) -> (element=w444:string)
          n152 = Set Menu Item Info(7:w444, 8:w441, 9:w439, 11:w443) -> (0:w440:errorcluster, 3:w442:refnum<k9>)  [unwired: 1 in, 2 out]
        }
        frame "English", Default {
          n153 = call "CRYGet Window Menu.vi"("Tags"=string[] ["APP_SC_EXPORT_SIMPLIFIED_IMAGE", "DA_EXPORT_DOCUMENT"]) -> ("Tags_Out"=w462:string[], "Names_Out"=w463:string[])  [unwired: 8 in, 1 out]
          n154 = Insert Menu Items(5:w466, 6:w461, 7:w462, 8:w463, 9:w465) -> (0:w455:errorcluster, 1:w459:string[], 3:w457:refnum<k9>)  [unwired: 1 out]
          n155 = Index Array(array=w459, index=1) -> (element=w458:string)
          n156 = Set Menu Item Info(7:w458, 8:w455, 9:w453, 11:w457) -> (0:w454:errorcluster, 3:w456:refnum<k9>)  [unwired: 1 in, 2 out]
        }
      }
      n157 = Merge Errors(w304, w303) -> (w302:errorcluster)
    }
    frame "XY" {
      (unwired) u8 2 ("y")
      w556 = string[] ["DA_SCALE_Y_A", "DA_SCALE_Y_L"]
      n158 = Delete Menu Items(9:w644) -> (0:w540:errorcluster, 3:w653:refnum<k9>)  [unwired: 1 in, 2 out]
      n159 = call "CRYGet Window Menu.vi"("Tags"=string[] ["DA_SHOW", "DA_GRAPH", "DA_AXIS", "DA_REMOVEALL", "APP_SEPARATOR", "DA_XSCALE", "DA_YSCALE", "APP_SEPARATOR", "DA_EXPORT", "APP_SEPARATOR", "DA_PROPERTY"]) -> ("Tags_Out"=w570:string[], "Names_Out"=w571:string[])  [unwired: 8 in, 1 out]
      n160 = Insert Menu Items(6:w540, 7:w570, 8:w571, 9:w653) -> (0:w539:errorcluster, 1:w651:string[], 3:w589:refnum<k9>)  [unwired: 1 in, 1 out]
      n161 = Select(t="DA_AXIS_PHA_HIDE", s=w493, f="DA_AXIS_PHA_VIEW") -> (s? t:f=w499:string)
      n162 = Select(t="DA_AXIS_MAG_HIDE", s=w492, f="DA_AXIS_MAG_VIEW") -> (s? t:f=w500:string)
      n163 = Select(t="DA_LEG_HIDE", s=w596, f="DA_LEG_VIEW") -> (s? t:f=w567:string)
      n164 = Build Array(w500, w499) -> (w503:string[])
      n165 = call "CRYGet Window Menu.vi"("Tags"=w503) -> ("Tags_Out"=w568:string[], "Names_Out"=w569:string[])  [unwired: 8 in, 1 out]
      n166 = Build Array(w567) -> (w566:string[])
      n167 = call "CRYGet Window Menu.vi"("Tags"=w566) -> ("Names_Out"=w565:string[])  [unwired: 8 in, 2 out]
      n168 = Index Array(array=w565) -> (element=w564:string)  [unwired: 1 in]
      n169 = Index Array(array=w651, index #1=0 ("index"), index #2=1 ("index"), index #3=2 ("index"), index #4=3 ("index"), index #5=4 ("index"), index #6=5 ("index"), index #7=6 ("index"), index #8=7 ("index"), index #9=8 ("index")) -> (element #1=w552:string, element #2=w585:string, element #3=w584:string, element #4=w577:string, element #6=w628:string, element #7=w629:string, element #9=w639:string)  [unwired: 2 out]
      n170 = Insert Menu Items(5:w552, 6:w539, 7:w567, 8:w564, 9:w589) -> (0:w538:errorcluster, 3:w643:refnum<k9>)  [unwired: 1 in, 1 out]
      n171 = Set Menu Item Info(6:w596, 7:w567, 8:w538, 9:TRUE ("enabled"), 10:w564, 11:w643) -> (0:w537:errorcluster, 3:w642:refnum<k9>)  [unwired: 1 out]
      n172 = Index Array(array=w568, index #1=0 ("index"), index #2=1 ("index")) -> (element #1=w587:string, element #2=w495:string)
      n173 = Select(t="DA_CUR_HIDE", s=w591, f="DA_CUR_VIEW") -> (s? t:f=w563:string)
      n174 = Build Array(w563) -> (w562:string[])
      n175 = call "CRYGet Window Menu.vi"("Tags"=w562) -> ("Names_Out"=w561:string[])  [unwired: 8 in, 2 out]
      n176 = Index Array(array=w561) -> (element=w560:string)  [unwired: 1 in]
      n177 = Insert Menu Items(5:w552, 6:w537, 7:w563, 8:w560, 9:w642) -> (0:w536:errorcluster, 3:w573:refnum<k9>)  [unwired: 2 out]
      n178 = Set Menu Item Info(6:w591, 7:w563, 8:w536, 9:w574, 10:w560, 11:w573) -> (0:w530:errorcluster)  [unwired: 2 out]
      n179 = Insert Menu Items(5:w584, 6:w530, 7:w568, 8:w569, 9:w589) -> (0:w529:errorcluster, 3:w586:refnum<k9>)  [unwired: 2 out]
      n180 = Set Menu Item Info(6:w492, 7:w587, 8:w529, 9:TRUE ("enabled"), 11:w586) -> (0:w497:errorcluster, 3:w494:refnum<k9>)  [unwired: 2 out]
      n181 = Set Menu Item Info(6:w493, 7:w495, 8:w497, 9:TRUE ("enabled"), 11:w494) -> (0:w496:errorcluster)  [unwired: 3 out]
      n182 = Set Menu Item Info(7:w577, 8:w496, 9:w575, 11:w573) -> (0:w527:errorcluster)  [unwired: 1 in, 3 out]
      n183 = disable-structure shown="Enabled" {
        disable-tunnel: w576 -> [w689 _]
        disable-tunnel: w574 -> [w688 _]
        disable-tunnel: w573 -> [w687 w694]
        disable-tunnel: [w682 w694] -> w553
        disable-tunnel: w552 -> [w681 _]
        disable-tunnel: [_ w693] -> w528
        disable-tunnel: w527 -> [_ w693]
        frame Disabled {
          n184 = Select(t="DA_PRE_HIDE", s=w689, f="DA_PRE_VIEW") -> (s? t:f=w684:string)
          n185 = Build Array(w684) -> (w685:string[])
          n186 = call "CRYGet Window Menu.vi"("Tags"=w685) -> ("Names_Out"=w686:string[])  [unwired: 8 in, 2 out]
          n187 = Index Array(array=w686) -> (element=w683:string)  [unwired: 1 in]
          n188 = Insert Menu Items(5:w681, 7:w684, 8:w683, 9:w687) -> (3:w690:refnum<k9>)  [unwired: 1 in, 3 out]
          n189 = Set Menu Item Info(6:w689, 7:w684, 9:w688, 10:w683, 11:w690) -> (3:w682:refnum<k9>)  [unwired: 1 in, 2 out]
        }
        frame Enabled {
        }
      }
      n190 = Select(t="DA_PAL_HIDE", s=w546, f="DA_PAL_VIEW") -> (s? t:f=w548:string)
      n191 = Build Array(w548) -> (w551:string[])
      n192 = call "CRYGet Window Menu.vi"("Tags"=w551) -> ("Names_Out"=w550:string[])  [unwired: 8 in, 2 out]
      n193 = Index Array(array=w550) -> (element=w547:string)  [unwired: 1 in]
      n194 = Insert Menu Items(5:w552, 6:w528, 7:w548, 8:w547, 9:w553) -> (0:w526:errorcluster, 3:w549:refnum<k9>)  [unwired: 2 out]
      n195 = Set Menu Item Info(6:w546, 7:w548, 8:w526, 10:w547, 11:w549) -> (0:w525:errorcluster)  [unwired: 1 in, 2 out]
      n196 = Insert Menu Items(5:w585, 6:w525, 7:w597, 8:w579, 9:w573) -> (0:w535:errorcluster, 1:w582:string[], 3:w581:refnum<k9>)  [unwired: 1 out]
      n197 = Index Array(array=w582, index #1=0 ("index"), index #2=1 ("index"), index #3=2 ("index"), index #4=3 ("index"), index #5=4 ("index")) -> (element #1=w609:string, element #2=w608:string, element #3=w607:string, element #4=w606:string, element #5=w513:string)
      n198 = for {
        N: 4 -> [_]
        tunnel: w582 -> [w700] mode=indexing
        tunnel: w579 -> [w699] mode=indexing
        tunnel: w578 -> [w698] mode=indexing
        shift-right: [w697] -> w580
        shift-left: w581 -> [w701]
        shift-right: [w695] -> w534
        shift-left: w535 -> [w696]
        n199 = Set Menu Item Info(7:w700, 8:w696, 9:w698, 10:w699, 11:w701) -> (0:w695:errorcluster, 3:w697:refnum<k9>)  [unwired: 1 in, 1 out]
      }
      n200 = Insert Menu Items(5:w609, 6:w534, 7:w602, 8:w598, 9:w580) -> (0:w533:errorcluster, 3:w605:refnum<k9>)  [unwired: 2 out]
      n201 = Insert Menu Items(5:w608, 6:w533, 7:w601, 8:w598, 9:w605) -> (0:w532:errorcluster, 3:w604:refnum<k9>)  [unwired: 2 out]
      n202 = Insert Menu Items(5:w607, 6:w532, 7:w600, 8:w598, 9:w604) -> (0:w531:errorcluster, 3:w603:refnum<k9>)  [unwired: 2 out]
      n203 = Insert Menu Items(5:w606, 6:w531, 7:w599, 8:w598, 9:w603) -> (0:w519:errorcluster, 3:w517:refnum<k9>)  [unwired: 2 out]
      n204 = Not(x=w515) -> (.not. x?=w520:bool)
      n205 = Equal?(x=w617, y=u8 1) -> (x = y?=w616:bool)
      n206 = Set Menu Item Info(7:w513, 8:w519, 9:w520, 11:w517) -> (0:w518:errorcluster, 3:w516:refnum<k9>)  [unwired: 1 in, 2 out]
      n207 = call "CRYGet Window Menu.vi"("Tags"=string[] ["DA_SCALE_X_A", "DA_SCALE_X_L"]) -> ("Tags_Out"=w557:string[], "Names_Out"=w558:string[])  [unwired: 8 in, 1 out]
      n208 = Index Array(array=w557, index #1=0 ("index"), index #2=1 ("index")) -> (element #1=w625:string, element #2=w624:string)
      n209 = Insert Menu Items(5:w628, 6:w518, 7:w557, 8:w558, 9:w516) -> (0:w521:errorcluster, 3:w638:refnum<k9>)  [unwired: 2 out]
      n210 = Equal?(x=w615, y=u8 1) -> (x = y?=w614:bool)
      n211 = Index Array(array=w556, index #1=0 ("index"), index #2=1 ("index")) -> (element #1=w621:string, element #2=w620:string)
      n212 = call "CRYGet Window Menu.vi"("Tags"=w556) -> ("Tags_Out"=w554:string[], "Names_Out"=w555:string[])  [unwired: 8 in, 1 out]
      n213 = Insert Menu Items(5:w629, 6:w521, 7:w554, 8:w555, 9:w638) -> (0:w488:errorcluster, 3:w636:refnum<k9>)  [unwired: 2 out]
      n214 = Set Menu Item Info(6:w543, 7:w625, 9:TRUE ("enabled"), 11:w636) -> (0:w524:errorcluster, 3:w635:refnum<k9>)  [unwired: 1 in, 2 out]
      n215 = Set Menu Item Info(6:w616, 7:w624, 8:w524, 9:TRUE ("enabled"), 11:w635) -> (0:w523:errorcluster, 3:w631:refnum<k9>)  [unwired: 2 out]
      n216 = Set Menu Item Info(6:w542, 7:w621, 8:w523, 9:TRUE ("enabled"), 11:w631) -> (0:w522:errorcluster, 3:w630:refnum<k9>)  [unwired: 2 out]
      n217 = Set Menu Item Info(6:w614, 7:w620, 8:w522, 9:TRUE ("enabled"), 11:w630) -> (0:w487:errorcluster)  [unwired: 3 out]
      n218 = case shown="\"Chinese\", \"Korean\"" w541 {
        tunnel: w639 -> [w667 w680]
        tunnel: w636 -> [w666 w679]
        tunnel: [w663 w676] -> w509
        tunnel: w575 -> [w662 w675]
        tunnel: w488 -> [w658 w671]
        tunnel: [w656 w670] -> w491
        tunnel: [2 ("index") 1 ("index")] -> w512
        tunnel: [w655 w668] -> w511
        frame "English", Default {
          n219 = call "CRYGet Window Menu.vi"("Tags"=string[] ["APP_SC_EXPORT_SIMPLIFIED_IMAGE", "DA_EXPORT_EXCEL", "DA_EXPORT_DOCUMENT"]) -> ("Tags_Out"=w659:string[], "Names_Out"=w660:string[])  [unwired: 8 in, 1 out]
          n220 = Insert Menu Items(5:w667, 6:w658, 7:w659, 8:w660, 9:w666) -> (0:w657:errorcluster, 1:w655:string[], 3:w663:refnum<k9>)  [unwired: 1 out]
          n221 = Index Array(array=w655, index=1) -> (element=w664:string)
          n222 = Set Menu Item Info(7:w664, 8:w657, 9:w662, 11:w663) -> (0:w656:errorcluster)  [unwired: 1 in, 3 out]
        }
        frame "Chinese", "Korean" {
          n223 = call "CRYGet Window Menu.vi"("Tags"=string[] ["DA_EXPORT_EXCEL", "DA_EXPORT_DOCUMENT"]) -> ("Tags_Out"=w672:string[], "Names_Out"=w673:string[])  [unwired: 8 in, 1 out]
          n224 = Insert Menu Items(5:w680, 6:w671, 7:w672, 8:w673, 9:w679) -> (0:w670:errorcluster, 1:w668:string[], 3:w676:refnum<k9>)  [unwired: 1 out]
          n225 = Index Array(array=w668, index=0) -> (element=w677:string)
          n226 = Set Menu Item Info(7:w677, 9:w675, 11:w676) -> ()  [unwired: 2 in, 4 out]
        }
      }
      n227 = Index Array(array=w511, index=w512) -> (element=w510:string)
      n228 = Set Menu Item Info(7:w510, 8:w487, 9:w508, 11:w509) -> (0:w490:errorcluster)  [unwired: 1 in, 3 out]
      n229 = Merge Errors(w491, w490) -> (w489:errorcluster)
    }
    frame "POLAR_XY" {
      (unwired) u8 2 ("y")
      w780 = string[] ["DA_SCALE_Y_A", "DA_SCALE_Y_L"]
      n230 = Delete Menu Items(9:w736) -> (0:w719:errorcluster, 3:w737:refnum<k9>)  [unwired: 1 in, 2 out]
      n231 = call "CRYGet Window Menu.vi"("Tags"=string[] ["DA_SHOW", "DA_REMOVEALL", "APP_SEPARATOR", "DA_XSCALE", "DA_YSCALE", "APP_SEPARATOR", "DA_EXPORT", "APP_SEPARATOR", "DA_PROPERTY"]) -> ("Tags_Out"=w772:string[], "Names_Out"=w771:string[])  [unwired: 8 in, 1 out]
      n232 = Insert Menu Items(6:w719, 7:w772, 8:w771, 9:w737) -> (0:w718:errorcluster, 1:w738:string[], 3:w769:refnum<k9>)  [unwired: 2 out]
      n233 = Select(t="DA_LEG_HIDE", s=w735, f="DA_LEG_VIEW") -> (s? t:f=w773:string)
      n234 = Build Array(w773) -> (w774:string[])
      n235 = call "CRYGet Window Menu.vi"("Tags"=w774) -> ("Names_Out"=w775:string[])  [unwired: 8 in, 2 out]
      n236 = Index Array(array=w775) -> (element=w776:string)  [unwired: 1 in]
      n237 = Index Array(array=w738, index #1=0 ("index"), index #2=1 ("index"), index #3=2 ("index"), index #4=3 ("index"), index #5=4 ("index"), index #6=5 ("index"), index #7=6 ("index")) -> (element #1=w783:string, element #2=w794:string, element #4=w795:string, element #5=w796:string, element #7=w728:string)  [unwired: 2 out]
      n238 = Insert Menu Items(5:w783, 6:w718, 7:w773, 8:w776, 9:w769) -> (0:w717:errorcluster, 3:w744:refnum<k9>)  [unwired: 1 in, 1 out]
      n239 = Set Menu Item Info(6:w735, 7:w773, 8:w717, 9:TRUE ("enabled"), 10:w776, 11:w744) -> (0:w716:errorcluster, 3:w791:refnum<k9>)  [unwired: 1 out]
      n240 = Select(t="DA_PAL_HIDE", s=w730, f="DA_PAL_VIEW") -> (s? t:f=w787:string)
      n241 = Build Array(w787) -> (w784:string[])
      n242 = call "CRYGet Window Menu.vi"("Tags"=w784) -> ("Names_Out"=w785:string[])  [unwired: 8 in, 2 out]
      n243 = Index Array(array=w785) -> (element=w788:string)  [unwired: 1 in]
      n244 = Insert Menu Items(5:w783, 6:w716, 7:w787, 8:w788, 9:w791) -> (0:w715:errorcluster, 3:w786:refnum<k9>)  [unwired: 2 out]
      n245 = Set Menu Item Info(6:w730, 7:w787, 8:w715, 10:w788, 11:w786) -> (0:w714:errorcluster)  [unwired: 1 in, 2 out]
      n246 = Set Menu Item Info(7:w794, 8:w714, 9:w726, 11:w791) -> (0:w713:errorcluster, 3:w792:refnum<k9>)  [unwired: 1 in, 2 out]
      n247 = Equal?(x=w732, y=u8 1) -> (x = y?=w764:bool)
      n248 = call "CRYGet Window Menu.vi"("Tags"=string[] ["DA_SCALE_X_A", "DA_SCALE_X_L"]) -> ("Tags_Out"=w779:string[], "Names_Out"=w778:string[])  [unwired: 8 in, 1 out]
      n249 = Index Array(array=w779, index #1=0 ("index"), index #2=1 ("index")) -> (element #1=w756:string, element #2=w757:string)
      n250 = Insert Menu Items(5:w795, 6:w713, 7:w779, 8:w778, 9:w792) -> (0:w709:errorcluster, 3:w746:refnum<k9>)  [unwired: 2 out]
      n251 = Equal?(x=w731, y=u8 1) -> (x = y?=w765:bool)
      n252 = Index Array(array=w780, index #1=0 ("index"), index #2=1 ("index")) -> (element #1=w760:string, element #2=w761:string)
      n253 = call "CRYGet Window Menu.vi"("Tags"=w780) -> ("Tags_Out"=w782:string[], "Names_Out"=w781:string[])  [unwired: 8 in, 1 out]
      n254 = Insert Menu Items(5:w796, 6:w709, 7:w782, 8:w781, 9:w746) -> (0:w707:errorcluster, 3:w725:refnum<k9>)  [unwired: 2 out]
      n255 = Set Menu Item Info(6:w734, 7:w756, 9:TRUE ("enabled"), 11:w725) -> (0:w712:errorcluster, 3:w748:refnum<k9>)  [unwired: 1 in, 2 out]
      n256 = Set Menu Item Info(6:w764, 7:w757, 8:w712, 9:TRUE ("enabled"), 11:w748) -> (0:w711:errorcluster, 3:w752:refnum<k9>)  [unwired: 2 out]
      n257 = Set Menu Item Info(6:w733, 7:w760, 8:w711, 9:TRUE ("enabled"), 11:w752) -> (0:w710:errorcluster, 3:w753:refnum<k9>)  [unwired: 2 out]
      n258 = Set Menu Item Info(6:w765, 7:w761, 8:w710, 9:TRUE ("enabled"), 11:w753) -> (0:w706:errorcluster)  [unwired: 3 out]
      n259 = case shown="\"Chinese\", \"Korean\"" w727 {
        tunnel: w728 -> [w816 w829]
        tunnel: w725 -> [w815 w828]
        tunnel: [w812 w825] -> w723
        tunnel: w726 -> [w811 w824]
        tunnel: [w806 w820] -> w722
        tunnel: [2 ("index") 1 ("index")] -> w721
        tunnel: [w804 w817] -> w708
        frame "English", Default {
          n260 = call "CRYGet Window Menu.vi"("Tags"=string[] ["APP_SC_EXPORT_SIMPLIFIED_IMAGE", "DA_EXPORT_EXCEL", "DA_EXPORT_DOCUMENT"]) -> ("Tags_Out"=w808:string[], "Names_Out"=w809:string[])  [unwired: 8 in, 1 out]
          n261 = Insert Menu Items(5:w816, 7:w808, 8:w809, 9:w815) -> (0:w805:errorcluster, 1:w806:string[], 3:w812:refnum<k9>)  [unwired: 1 in, 1 out]
          n262 = Index Array(array=w806, index=1) -> (element=w813:string)
          n263 = Set Menu Item Info(7:w813, 8:w805, 9:w811, 11:w812) -> (0:w804:errorcluster)  [unwired: 1 in, 3 out]
        }
        frame "Chinese", "Korean" {
          n264 = call "CRYGet Window Menu.vi"("Tags"=string[] ["DA_EXPORT_EXCEL", "DA_EXPORT_DOCUMENT"]) -> ("Tags_Out"=w821:string[], "Names_Out"=w822:string[])  [unwired: 8 in, 1 out]
          n265 = Insert Menu Items(5:w829, 7:w821, 8:w822, 9:w828) -> (0:w818:errorcluster, 1:w820:string[], 3:w825:refnum<k9>)  [unwired: 1 in, 1 out]
          n266 = Index Array(array=w820, index=0) -> (element=w826:string)
          n267 = Set Menu Item Info(7:w826, 8:w818, 9:w824, 11:w825) -> (0:w817:errorcluster)  [unwired: 1 in, 3 out]
        }
      }
      n268 = Index Array(array=w722, index=w721) -> (element=w724:string)
      n269 = Set Menu Item Info(7:w724, 8:w708, 9:w720, 11:w723) -> (0:w705:errorcluster)  [unwired: 1 in, 3 out]
      n270 = call "CRYGet Window Menu.vi"("Tags"=string[] ["APP_SEPARATOR"] ("item tags")) -> ("Tags_Out"=w800:string[], "Names_Out"=w799:string[])  [unwired: 8 in, 1 out]
      n271 = Insert Menu Items(6:w705, 7:w800, 8:w799, 9:w723) -> (0:w704:errorcluster, 3:w797:refnum<k9>)  [unwired: 3 out]
      n272 = call "CRYGet Window Menu.vi"("Tags"=string[] ["DA_XY_HIDE_1"]) -> ("Tags_Out"=w803:string[], "Names_Out"=w802:string[])  [unwired: 8 in, 1 out]
      n273 = Insert Menu Items(6:w704, 7:w803, 8:w802, 9:w797) -> (0:w703:errorcluster, 3:w729:refnum<k9>)  [unwired: 3 out]
      n274 = Merge Errors(w703, w707, w706) -> (w702:errorcluster)
    }
    frame "DIGITAL" {
      n275 = Delete Menu Items(9:w950) -> (0:w863:errorcluster, 3:w960:refnum<k9>)  [unwired: 1 in, 2 out]
      n276 = call "CRYGet Window Menu.vi"("Tags"=string[] ["DA_SHOW", "DA_GRAPH", "DA_REMOVEALL", "APP_SEPARATOR", "DA_XSCALE", "DA_YSCALE", "APP_SEPARATOR", "DA_EXPORT", "APP_SEPARATOR", "DA_PROPERTY"]) -> ("Tags_Out"=w888:string[], "Names_Out"=w887:string[])  [unwired: 8 in, 1 out]
      n277 = Insert Menu Items(6:w863, 7:w888, 8:w887, 9:w960) -> (0:w862:errorcluster, 1:w958:string[], 3:w949:refnum<k9>)  [unwired: 2 out]
      n278 = Select(t="DA_LEG_HIDE", s=w902, f="DA_LEG_VIEW") -> (s? t:f=w886:string)
      n279 = Build Array(w886) -> (w885:string[])
      n280 = call "CRYGet Window Menu.vi"("Tags"=w885) -> ("Names_Out"=w884:string[])  [unwired: 8 in, 2 out]
      n281 = Index Array(array=w884) -> (element=w883:string)  [unwired: 1 in]
      n282 = Index Array(array=w958, index #1=0 ("index"), index #2=1 ("index"), index #3=2 ("index"), index #4=3 ("index"), index #5=4 ("index"), index #6=5 ("index"), index #7=6 ("index"), index #8=7 ("index")) -> (element #1=w868:string, element #2=w951:string, element #3=w892:string, element #5=w934:string, element #6=w935:string, element #8=w944:string)  [unwired: 2 out]
      n283 = Insert Menu Items(5:w868, 6:w862, 7:w886, 8:w883, 9:w949) -> (0:w861:errorcluster, 3:w948:refnum<k9>)  [unwired: 1 in, 1 out]
      n284 = Set Menu Item Info(6:w902, 7:w886, 8:w861, 9:TRUE ("enabled"), 10:w883, 11:w948) -> (0:w860:errorcluster, 3:w947:refnum<k9>)  [unwired: 1 out]
      n285 = disable-structure shown="Enabled" {
        disable-tunnel: w947 -> [w1004 w1005]
        disable-tunnel: w868 -> [w1003 _]
        disable-tunnel: [w1001 w1005] -> w869
        disable-tunnel: w899 -> [w998 _]
        frame Disabled {
          w996 = "Cursor"
          n286 = Select(t="DA_CUR_HIDE", s=w998, f="DA_CUR_VIEW") -> (s? t:f=w997:string)
          n287 = Insert Menu Items(5:w1003, 7:w997, 8:w996, 9:w1004) -> (3:w1001:refnum<k9>)  [unwired: 1 in, 3 out]
          n288 = Set Menu Item Info(6:w998, 7:w997, 9:TRUE ("enabled"), 10:w996, 11:w1001) -> ()  [unwired: 1 in, 3 out]
        }
        frame Enabled {
        }
      }
      n289 = Select(t="DA_PAL_HIDE", s=w867, f="DA_PAL_VIEW") -> (s? t:f=w873:string)
      n290 = Build Array(w873) -> (w876:string[])
      n291 = call "CRYGet Window Menu.vi"("Tags"=w876) -> ("Names_Out"=w875:string[])  [unwired: 8 in, 2 out]
      n292 = Index Array(array=w875) -> (element=w872:string)  [unwired: 1 in]
      n293 = Set Menu Item Info(7:w892, 8:w860, 9:w890, 11:w869) -> (0:w859:errorcluster)  [unwired: 1 in, 3 out]
      n294 = Insert Menu Items(5:w868, 6:w859, 7:w873, 8:w872, 9:w869) -> (0:w858:errorcluster, 3:w874:refnum<k9>)  [unwired: 2 out]
      n295 = Set Menu Item Info(7:w873, 8:w858, 10:w872, 11:w874) -> (0:w857:errorcluster)  [unwired: 2 in, 2 out]
      n296 = Insert Menu Items(5:w951, 6:w857, 7:w903, 8:w896, 9:w869) -> (0:w856:errorcluster, 1:w897:string[], 3:w894:refnum<k9>)  [unwired: 1 out]
      n297 = Index Array(array=w897, index #1=0 ("index"), index #2=1 ("index"), index #3=2 ("index"), index #4=3 ("index"), index #5=4 ("index")) -> (element #1=w915:string, element #2=w914:string, element #3=w913:string, element #4=w912:string, element #5=w840:string)
      n298 = for {
        N: 4 -> [_]
        tunnel: w897 -> [w994] mode=indexing
        tunnel: w896 -> [w993] mode=indexing
        tunnel: w895 -> [w992] mode=indexing
        shift-right: [w991] -> w893
        shift-left: w894 -> [w995]
        shift-right: [w989] -> w855
        shift-left: w856 -> [w990]
        n299 = Set Menu Item Info(7:w994, 8:w990, 9:w992, 10:w993, 11:w995) -> (0:w989:errorcluster, 3:w991:refnum<k9>)  [unwired: 1 in, 1 out]
      }
      n300 = Insert Menu Items(5:w915, 6:w855, 7:w908, 8:w904, 9:w893) -> (0:w854:errorcluster, 3:w911:refnum<k9>)  [unwired: 2 out]
      n301 = Insert Menu Items(5:w914, 6:w854, 7:w907, 8:w904, 9:w911) -> (0:w853:errorcluster, 3:w910:refnum<k9>)  [unwired: 2 out]
      n302 = Insert Menu Items(5:w913, 6:w853, 7:w906, 8:w904, 9:w910) -> (0:w852:errorcluster, 3:w909:refnum<k9>)  [unwired: 2 out]
      n303 = Insert Menu Items(5:w912, 6:w852, 7:w905, 8:w904, 9:w909) -> (0:w844:errorcluster, 3:w846:refnum<k9>)  [unwired: 2 out]
      n304 = Not(x=w842) -> (.not. x?=w847:bool)
      n305 = Set Menu Item Info(7:w840, 8:w844, 9:w847, 11:w846) -> (0:w843:errorcluster, 3:w845:refnum<k9>)  [unwired: 1 in, 2 out]
      n306 = call "CRYGet Window Menu.vi"("Tags"=string[] ["DA_SCALE_X_A", "DA_SCALE_X_L"]) -> ("Tags_Out"=w880:string[], "Names_Out"=w882:string[])  [unwired: 8 in, 1 out]
      n307 = Equal?(x=w923, y=u8 1) -> (x = y?=w922:bool)
      n308 = Index Array(array=w880, index #1=0 ("index"), index #2=1 ("index")) -> (element #1=w931:string, element #2=w930:string)
      n309 = Insert Menu Items(5:w934, 6:w843, 7:w880, 8:w882, 9:w845) -> (0:w851:errorcluster, 3:w943:refnum<k9>)  [unwired: 2 out]
      n310 = Equal?(x=w921, y=u8 1) -> (x = y?=w920:bool)
      n311 = call "CRYGet Window Menu.vi"("Tags"=string[] ["DA_SCALE_Y_A", "DA_SCALE_Y_L"]) -> ("Tags_Out"=w878:string[], "Names_Out"=w877:string[])  [unwired: 8 in, 1 out]
      n312 = Insert Menu Items(5:w935, 6:w851, 7:w878, 8:w877, 9:w943) -> (0:w834:errorcluster, 3:w891:refnum<k9>)  [unwired: 2 out]
      n313 = Set Menu Item Info(6:w866, 7:w931, 9:TRUE ("enabled"), 11:w891) -> (0:w850:errorcluster, 3:w941:refnum<k9>)  [unwired: 1 in, 2 out]
      n314 = Set Menu Item Info(6:w922, 7:w930, 8:w850, 9:TRUE ("enabled"), 11:w941) -> (0:w849:errorcluster, 3:w937:refnum<k9>)  [unwired: 2 out]
      n315 = Index Array(array=w878, index #1=0 ("index"), index #2=1 ("index")) -> (element #1=w927:string, element #2=w926:string)
      n316 = Set Menu Item Info(6:w865, 7:w927, 8:w849, 9:TRUE ("enabled"), 11:w937) -> (0:w848:errorcluster, 3:w936:refnum<k9>)  [unwired: 2 out]
      n317 = Set Menu Item Info(6:w920, 7:w926, 8:w848, 9:TRUE ("enabled"), 11:w936) -> (0:w833:errorcluster)  [unwired: 3 out]
      n318 = case shown="\"English\", Default" w864 {
        tunnel: w944 -> [w974 w988]
        tunnel: w891 -> [w973 w987]
        tunnel: [w972 w986] -> w838
        tunnel: w890 -> [w971 w985]
        tunnel: w834 -> [w965 w979]
        tunnel: [w963 w977] -> w832
        tunnel: [w962 w976] -> w837
        tunnel: [1 ("index") 2 ("index")] -> w836
        frame "Chinese", "Korean" {
          n319 = call "CRYGet Window Menu.vi"("Tags"=string[] ["DA_EXPORT_EXCEL", "DA_EXPORT_DOCUMENT"]) -> ("Tags_Out"=w967:string[], "Names_Out"=w966:string[])  [unwired: 8 in, 1 out]
          n320 = Insert Menu Items(5:w974, 6:w965, 7:w967, 8:w966, 9:w973) -> (0:w964:errorcluster, 1:w962:string[], 3:w972:refnum<k9>)  [unwired: 1 out]
          n321 = Index Array(array=w962, index=0) -> (element=w969:string)
          n322 = Set Menu Item Info(7:w969, 8:w964, 9:w971, 11:w972) -> (0:w963:errorcluster)  [unwired: 1 in, 3 out]
        }
        frame "English", Default {
          n323 = call "CRYGet Window Menu.vi"("Tags"=string[] ["APP_SC_EXPORT_SIMPLIFIED_IMAGE", "DA_EXPORT_EXCEL", "DA_EXPORT_DOCUMENT"]) -> ("Tags_Out"=w981:string[], "Names_Out"=w980:string[])  [unwired: 8 in, 1 out]
          n324 = Insert Menu Items(5:w988, 6:w979, 7:w981, 8:w980, 9:w987) -> (0:w978:errorcluster, 1:w976:string[], 3:w986:refnum<k9>)  [unwired: 1 out]
          n325 = Index Array(array=w976, index=1) -> (element=w983:string)
          n326 = Set Menu Item Info(7:w983, 8:w978, 9:w985, 11:w986) -> (0:w977:errorcluster)  [unwired: 1 in, 3 out]
        }
      }
      n327 = Index Array(array=w837, index=w836) -> (element=w839:string)
      n328 = Set Menu Item Info(7:w839, 8:w833, 9:w835, 11:w838) -> (0:w831:errorcluster)  [unwired: 1 in, 3 out]
      n329 = Merge Errors(w832, w831) -> (w830:errorcluster)
    }
    frame "OCTAVE" {
      n330 = Delete Menu Items(9:w1136) -> (0:w1041:errorcluster, 3:w1146:refnum<k9>)  [unwired: 1 in, 2 out]
      n331 = call "CRYGet Window Menu.vi"("Tags"=string[] ["DA_SHOW", "DA_GRAPH", "DA_REMOVEALL", "APP_SEPARATOR", "DA_XSCALE", "DA_YSCALE", "APP_SEPARATOR", "DA_EXPORT", "APP_SEPARATOR", "DA_PROPERTY"]) -> ("Tags_Out"=w1069:string[], "Names_Out"=w1071:string[])  [unwired: 8 in, 1 out]
      n332 = Insert Menu Items(6:w1041, 7:w1069, 8:w1071, 9:w1146) -> (0:w1040:errorcluster, 1:w1144:string[], 3:w1135:refnum<k9>)  [unwired: 2 out]
      n333 = Select(t="DA_LEG_HIDE", s=w1088, f="DA_LEG_VIEW") -> (s? t:f=w1066:string)
      n334 = Build Array(w1066) -> (w1068:string[])
      n335 = call "CRYGet Window Menu.vi"("Tags"=w1068) -> ("Names_Out"=w1067:string[])  [unwired: 8 in, 2 out]
      n336 = Index Array(array=w1067) -> (element=w1065:string)  [unwired: 1 in]
      n337 = Index Array(array=w1144, index #1=0 ("index"), index #2=1 ("index"), index #3=2 ("index"), index #4=3 ("index"), index #5=4 ("index"), index #6=5 ("index"), index #7=6 ("index"), index #8=7 ("index")) -> (element #1=w1046:string, element #2=w1137:string, element #3=w1078:string, element #5=w1120:string, element #6=w1121:string, element #8=w1130:string)  [unwired: 2 out]
      n338 = Insert Menu Items(5:w1046, 6:w1040, 7:w1066, 8:w1065, 9:w1135) -> (0:w1039:errorcluster, 3:w1134:refnum<k9>)  [unwired: 1 in, 1 out]
      n339 = Set Menu Item Info(6:w1088, 7:w1066, 8:w1039, 9:TRUE ("enabled"), 10:w1065, 11:w1134) -> (0:w1038:errorcluster, 3:w1133:refnum<k9>)  [unwired: 1 out]
      n340 = Select(t="DA_PAL_HIDE", s=w1047, f="DA_PAL_VIEW") -> (s? t:f=w1051:string)
      n341 = Build Array(w1051) -> (w1054:string[])
      n342 = Select(t="DA_CUR_HIDE", s=w1085, f="DA_CUR_VIEW") -> (s? t:f=w1062:string)
      n343 = call "CRYGet Window Menu.vi"("Tags"=w1054) -> ("Names_Out"=w1053:string[])  [unwired: 8 in, 2 out]
      n344 = Build Array(w1062) -> (w1064:string[])
      n345 = Index Array(array=w1053) -> (element=w1050:string)  [unwired: 1 in]
      n346 = call "CRYGet Window Menu.vi"("Tags"=w1064) -> ("Names_Out"=w1063:string[])  [unwired: 8 in, 2 out]
      n347 = Index Array(array=w1063) -> (element=w1061:string)  [unwired: 1 in]
      n348 = Insert Menu Items(5:w1046, 6:w1038, 7:w1062, 8:w1061, 9:w1133) -> (0:w1037:errorcluster, 3:w1077:refnum<k9>)  [unwired: 2 out]
      n349 = Set Menu Item Info(6:w1085, 7:w1062, 8:w1037, 9:w1072, 10:w1061, 11:w1077) -> (0:w1036:errorcluster, 3:w1045:refnum<k9>)  [unwired: 1 out]
      n350 = Insert Menu Items(5:w1046, 6:w1036, 7:w1051, 8:w1050, 9:w1045) -> (0:w1035:errorcluster, 3:w1052:refnum<k9>)  [unwired: 2 out]
      n351 = Set Menu Item Info(6:w1047, 7:w1051, 8:w1035, 10:w1050, 11:w1052) -> (0:w1034:errorcluster)  [unwired: 1 in, 2 out]
      n352 = Set Menu Item Info(7:w1078, 8:w1034, 9:w1075, 11:w1077) -> (0:w1033:errorcluster)  [unwired: 1 in, 3 out]
      n353 = Insert Menu Items(5:w1137, 6:w1033, 7:w1089, 8:w1082, 9:w1077) -> (0:w1032:errorcluster, 1:w1083:string[], 3:w1080:refnum<k9>)  [unwired: 1 out]
      n354 = Index Array(array=w1083, index #1=0 ("index"), index #2=1 ("index"), index #3=2 ("index"), index #4=3 ("index"), index #5=4 ("index")) -> (element #1=w1101:string, element #2=w1100:string, element #3=w1099:string, element #4=w1098:string, element #5=w1018:string)
      n355 = for {
        N: 4 -> [_]
        tunnel: w1083 -> [w1180] mode=indexing
        tunnel: w1082 -> [w1179] mode=indexing
        tunnel: w1081 -> [w1178] mode=indexing
        shift-right: [w1177] -> w1079
        shift-left: w1080 -> [w1181]
        shift-right: [w1175] -> w1031
        shift-left: w1032 -> [w1176]
        n356 = Set Menu Item Info(7:w1180, 8:w1176, 9:w1178, 10:w1179, 11:w1181) -> (0:w1175:errorcluster, 3:w1177:refnum<k9>)  [unwired: 1 in, 1 out]
      }
      n357 = Insert Menu Items(5:w1101, 6:w1031, 7:w1094, 8:w1090, 9:w1079) -> (0:w1030:errorcluster, 3:w1097:refnum<k9>)  [unwired: 2 out]
      n358 = Insert Menu Items(5:w1100, 6:w1030, 7:w1093, 8:w1090, 9:w1097) -> (0:w1029:errorcluster, 3:w1096:refnum<k9>)  [unwired: 2 out]
      n359 = Insert Menu Items(5:w1099, 6:w1029, 7:w1092, 8:w1090, 9:w1096) -> (0:w1028:errorcluster, 3:w1095:refnum<k9>)  [unwired: 2 out]
      n360 = Insert Menu Items(5:w1098, 6:w1028, 7:w1091, 8:w1090, 9:w1095) -> (0:w1017:errorcluster, 3:w1022:refnum<k9>)  [unwired: 2 out]
      n361 = Not(x=w1020) -> (.not. x?=w1023:bool)
      n362 = Set Menu Item Info(7:w1018, 8:w1017, 9:w1023, 11:w1022) -> (0:w1016:errorcluster, 3:w1021:refnum<k9>)  [unwired: 2 in, 1 out]
      n363 = call "CRYGet Window Menu.vi"("Tags"=string[] ["DA_SCALE_X_A", "DA_SCALE_X_L"]) -> ("Tags_Out"=w1058:string[], "Names_Out"=w1059:string[])  [unwired: 8 in, 1 out]
      n364 = Equal?(x=w1109, y=u8 1) -> (x = y?=w1108:bool)
      n365 = Index Array(array=w1058, index #1=0 ("index"), index #2=1 ("index")) -> (element #1=w1117:string, element #2=w1116:string)
      n366 = Insert Menu Items(5:w1120, 6:w1016, 7:w1058, 8:w1059, 9:w1021) -> (0:w1027:errorcluster, 3:w1129:refnum<k9>)  [unwired: 2 out]
      n367 = Equal?(x=w1107, y=u8 1) -> (x = y?=w1106:bool)
      n368 = call "CRYGet Window Menu.vi"("Tags"=string[] ["DA_SCALE_Y_A", "DA_SCALE_Y_L"]) -> ("Tags_Out"=w1055:string[], "Names_Out"=w1056:string[])  [unwired: 8 in, 1 out]
      n369 = Index Array(array=w1055, index #1=0 ("index"), index #2=1 ("index")) -> (element #1=w1113:string, element #2=w1112:string)
      n370 = Insert Menu Items(5:w1121, 6:w1027, 7:w1055, 8:w1056, 9:w1129) -> (0:w1010:errorcluster, 3:w1076:refnum<k9>)  [unwired: 2 out]
      n371 = Set Menu Item Info(6:w1044, 7:w1117, 9:TRUE ("enabled"), 11:w1076) -> (0:w1026:errorcluster, 3:w1127:refnum<k9>)  [unwired: 1 in, 2 out]
      n372 = Set Menu Item Info(6:w1108, 7:w1116, 8:w1026, 9:TRUE ("enabled"), 11:w1127) -> (0:w1025:errorcluster, 3:w1123:refnum<k9>)  [unwired: 2 out]
      n373 = Set Menu Item Info(6:w1043, 7:w1113, 8:w1025, 9:TRUE ("enabled"), 11:w1123) -> (0:w1024:errorcluster, 3:w1122:refnum<k9>)  [unwired: 2 out]
      n374 = Set Menu Item Info(6:w1106, 7:w1112, 8:w1024, 9:TRUE ("enabled"), 11:w1122) -> (0:w1009:errorcluster)  [unwired: 3 out]
      n375 = case shown="\"Chinese\", \"Korean\"" w1042 {
        tunnel: w1130 -> [w1160 w1174]
        tunnel: w1076 -> [w1159 w1173]
        tunnel: [w1158 w1172] -> w1014
        tunnel: w1075 -> [w1157 w1171]
        tunnel: w1010 -> [w1151 w1165]
        tunnel: [w1149 w1163] -> w1008
        tunnel: [w1147 w1162] -> w1013
        tunnel: [2 ("index") 1 ("index")] -> w1012
        frame "English", Default {
          n376 = call "CRYGet Window Menu.vi"("Tags"=string[] ["APP_SC_EXPORT_SIMPLIFIED_IMAGE", "DA_EXPORT_EXCEL", "DA_EXPORT_DOCUMENT"]) -> ("Tags_Out"=w1152:string[], "Names_Out"=w1153:string[])  [unwired: 8 in, 1 out]
          n377 = Insert Menu Items(5:w1160, 6:w1151, 7:w1152, 8:w1153, 9:w1159) -> (0:w1150:errorcluster, 1:w1147:string[], 3:w1158:refnum<k9>)  [unwired: 1 out]
          n378 = Index Array(array=w1147, index=1) -> (element=w1155:string)
          n379 = Set Menu Item Info(7:w1155, 8:w1150, 9:w1157, 11:w1158) -> (0:w1149:errorcluster)  [unwired: 1 in, 3 out]
        }
        frame "Chinese", "Korean" {
          n380 = call "CRYGet Window Menu.vi"("Tags"=string[] ["DA_EXPORT_EXCEL", "DA_EXPORT_DOCUMENT"]) -> ("Tags_Out"=w1166:string[], "Names_Out"=w1167:string[])  [unwired: 8 in, 1 out]
          n381 = Insert Menu Items(5:w1174, 6:w1165, 7:w1166, 8:w1167, 9:w1173) -> (0:w1164:errorcluster, 1:w1162:string[], 3:w1172:refnum<k9>)  [unwired: 1 out]
          n382 = Index Array(array=w1162, index=0) -> (element=w1169:string)
          n383 = Set Menu Item Info(7:w1169, 8:w1164, 9:w1171, 11:w1172) -> (0:w1163:errorcluster)  [unwired: 1 in, 3 out]
        }
      }
      n384 = Index Array(array=w1013, index=w1012) -> (element=w1015:string)
      n385 = Set Menu Item Info(7:w1015, 8:w1009, 9:w1011, 11:w1014) -> (0:w1007:errorcluster)  [unwired: 1 in, 3 out]
      n386 = Merge Errors(w1008, w1007) -> (w1006:errorcluster)
    }
    frame "POLAR" {
      n387 = Delete Menu Items(9:w1273) -> (0:w1233:errorcluster, 3:w1283:refnum<k9>)  [unwired: 1 in, 2 out]
      n388 = call "CRYGet Window Menu.vi"("Tags"=string[] ["DA_SHOW", "DA_GRAPH", "DA_REMOVEALL", "APP_SEPARATOR", "DA_EXPORT", "APP_SEPARATOR", "DA_PROPERTY"]) -> ("Tags_Out"=w1236:string[], "Names_Out"=w1237:string[])  [unwired: 8 in, 1 out]
      n389 = Insert Menu Items(6:w1233, 7:w1236, 8:w1237, 9:w1283) -> (0:w1232:errorcluster, 1:w1281:string[], 3:w1272:refnum<k9>)  [unwired: 2 out]
      n390 = Select(t="DA_FREQ_HIDE", s=w1214, f="DA_FREQ_VIEW") -> (s? t:f=w1240:string)
      n391 = Build Array(w1240) -> (w1242:string[])
      n392 = call "CRYGet Window Menu.vi"("Tags"=w1242) -> ("Names_Out"=w1241:string[])  [unwired: 8 in, 2 out]
      n393 = Index Array(array=w1241) -> (element=w1239:string)  [unwired: 1 in]
      n394 = Index Array(array=w1281, index #1=0 ("index"), index #2=1 ("index"), index #3=2 ("index"), index #4=3 ("index"), index #5=4 ("index"), index #6=5 ("index"), index #7=6 ("index")) -> (element #1=w1218:string, element #2=w1274:string, element #3=w1244:string, element #5=w1243:string, element #7=w1206:string)  [unwired: 2 out]
      n395 = Insert Menu Items(5:w1218, 6:w1232, 7:w1240, 8:w1239, 9:w1272) -> (0:w1231:errorcluster, 3:w1271:refnum<k9>)  [unwired: 1 in, 1 out]
      n396 = Set Menu Item Info(6:w1214, 7:w1240, 8:w1231, 9:TRUE ("enabled"), 10:w1239, 11:w1271) -> (0:w1213:errorcluster, 3:w1217:refnum<k9>)  [unwired: 1 out]
      n397 = Select(t="DA_XY_HIDE", s=w1215, f="DA_XY_VIEW") -> (s? t:f=w1225:string)
      n398 = Build Array(w1225) -> (w1221:string[])
      n399 = call "CRYGet Window Menu.vi"("Tags"=w1221) -> ("Names_Out"=w1220:string[])  [unwired: 8 in, 2 out]
      n400 = Index Array(array=w1220) -> (element=w1219:string)  [unwired: 1 in]
      n401 = Insert Menu Items(5:w1218, 6:w1213, 7:w1225, 8:w1219, 9:w1217) -> (0:w1212:errorcluster, 3:w1216:refnum<k9>)  [unwired: 1 in, 1 out]
      n402 = Set Menu Item Info(6:w1215, 7:w1225, 8:w1212, 9:TRUE ("enabled"), 10:w1219, 11:w1216) -> (0:w1211:errorcluster, 3:w1210:refnum<k9>)  [unwired: 1 out]
      n403 = Set Menu Item Info(7:w1244, 8:w1211, 9:w1189, 11:w1210) -> (0:w1196:errorcluster, 3:w1197:refnum<k9>)  [unwired: 1 in, 2 out]
      n404 = Not(x=w1200) -> (.not. x?=w1207:bool)
      n405 = Set Menu Item Info(7:w1206, 8:w1196, 9:w1207, 11:w1197) -> (0:w1209:errorcluster, 3:w1208:refnum<k9>)  [unwired: 1 in, 2 out]
      n406 = Insert Menu Items(5:w1274, 6:w1209, 7:w1253, 8:w1246, 9:w1208) -> (0:w1230:errorcluster, 1:w1249:string[], 3:w1248:refnum<k9>)  [unwired: 1 out]
      n407 = Index Array(array=w1249, index #1=0 ("index"), index #2=1 ("index"), index #3=2 ("index"), index #4=3 ("index"), index #5=4 ("index")) -> (element #1=w1265:string, element #2=w1264:string, element #3=w1263:string, element #4=w1262:string, element #5=w1198:string)
      n408 = for {
        N: 4 -> [_]
        tunnel: w1249 -> [w1289] mode=indexing
        tunnel: w1246 -> [w1288] mode=indexing
        tunnel: w1245 -> [w1287] mode=indexing
        shift-right: [w1286] -> w1247
        shift-left: w1248 -> [w1290]
        shift-right: [w1284] -> w1229
        shift-left: w1230 -> [w1285]
        n409 = Set Menu Item Info(7:w1289, 8:w1285, 9:w1287, 10:w1288, 11:w1290) -> (0:w1284:errorcluster, 3:w1286:refnum<k9>)  [unwired: 1 in, 1 out]
      }
      n410 = Insert Menu Items(5:w1265, 6:w1229, 7:w1258, 8:w1254, 9:w1247) -> (0:w1228:errorcluster, 3:w1261:refnum<k9>)  [unwired: 2 out]
      n411 = Insert Menu Items(5:w1264, 6:w1228, 7:w1257, 8:w1254, 9:w1261) -> (0:w1227:errorcluster, 3:w1260:refnum<k9>)  [unwired: 2 out]
      n412 = Insert Menu Items(5:w1263, 6:w1227, 7:w1256, 8:w1254, 9:w1260) -> (0:w1226:errorcluster, 3:w1259:refnum<k9>)  [unwired: 2 out]
      n413 = Insert Menu Items(5:w1262, 6:w1226, 7:w1255, 8:w1254, 9:w1259) -> (0:w1202:errorcluster, 3:w1204:refnum<k9>)  [unwired: 2 out]
      n414 = Not(x=w1200) -> (.not. x?=w1205:bool)
      n415 = Set Menu Item Info(7:w1198, 8:w1202, 9:w1205, 11:w1204) -> (0:w1201:errorcluster, 3:w1203:refnum<k9>)  [unwired: 1 in, 2 out]
      n416 = call "CRYGet Window Menu.vi"("Tags"=string[] ["DA_EXPORT_EXCEL", "DA_EXPORT_DOCUMENT"]) -> ("Tags_Out"=w1193:string[], "Names_Out"=w1234:string[])  [unwired: 8 in, 1 out]
      n417 = Insert Menu Items(5:w1243, 6:w1201, 7:w1193, 8:w1234, 9:w1203) -> (0:w1192:errorcluster, 1:w1190:string[], 3:w1191:refnum<k9>)  [unwired: 1 out]
      n418 = Index Array(array=w1190, index #1=0 ("index"), index #2=1 ("index")) -> (element #1=w1194:string, element #2=w1187:string)
      n419 = Set Menu Item Info(7:w1194, 8:w1192, 9:w1189, 11:w1191) -> (0:w1186:errorcluster, 3:w1185:refnum<k9>)  [unwired: 1 in, 2 out]
      n420 = Set Menu Item Info(7:w1187, 8:w1186, 9:w1182, 11:w1185) -> (0:w1183:errorcluster, 3:w1184:refnum<k9>)  [unwired: 1 in, 2 out]
    }
    frame "TABLE" {
      n421 = Delete Menu Items(9:w1372) -> (0:w1323:errorcluster, 3:w1373:refnum<k9>)  [unwired: 1 in, 2 out]
      n422 = call "CRYGet Window Menu.vi"("Tags"=string[] ["DA_GRAPH", "DA_REMOVESEL", "DA_REMOVEONE", "DA_REMOVEALL", "APP_SEPARATOR", "DA_EXPORT", "APP_SEPARATOR", "DA_PROPERTY"]) -> ("Tags_Out"=w1340:string[], "Names_Out"=w1341:string[])  [unwired: 8 in, 1 out]
      n423 = Variant To Data(type=refnum<vi> refnum ("WaveGraph Ref"), Variant=w1328) -> (data=w1330:refnum<vi>)  [unwired: 1 in, 1 out]
      n424 = Insert Menu Items(6:w1323, 7:w1340, 8:w1341, 9:w1373) -> (0:w1322:errorcluster, 1:w1368:string[], 3:w1306:refnum<k9>)  [unwired: 2 out]
      n425 = property class="Tbl"(reference=w1330) -> ("Selection Size"=w1327:T3)  [unwired: 1 in, 2 out]
      n426 = Unbundle By Name(w1327) -> ("Row"=w1326:i32)
      n427 = Index Array(array=w1368, index #1=0 ("index"), index #2=1 ("index"), index #3=2 ("index"), index #4=3 ("index"), index #5=5 ("index")) -> (element #1=w1365:string, element #2=w1334:string, element #3=w1333:string, element #4=w1331:string, element #5=w1332:string)
      n428 = Not Equal?(x=w1326, y=0) -> (x != y?=w1324:bool)
      n429 = Set Menu Item Info(7:w1334, 8:w1322, 9:w1324, 11:w1306) -> (0:w1321:errorcluster, 3:w1335:refnum<k9>)  [unwired: 1 in, 2 out]
      n430 = Set Menu Item Info(7:w1333, 8:w1321, 9:w1298, 11:w1335) -> (0:w1320:errorcluster, 3:w1343:refnum<k9>)  [unwired: 1 in, 2 out]
      n431 = Set Menu Item Info(7:w1331, 8:w1320, 9:w1298, 11:w1343) -> (0:w1304:errorcluster, 3:w1305:refnum<k9>)  [unwired: 1 in, 2 out]
      n432 = Insert Menu Items(5:w1365, 6:w1304, 7:w1360, 8:w1347, 9:w1305) -> (0:w1319:errorcluster, 1:w1348:string[], 3:w1350:refnum<k9>)  [unwired: 1 out]
      n433 = Index Array(array=w1348, index #1=0 ("index"), index #2=1 ("index"), index #3=2 ("index"), index #4=3 ("index"), index #5=4 ("index")) -> (element #1=w1354:string, element #2=w1353:string, element #3=w1352:string, element #4=w1351:string, element #5=w1308:string)
      n434 = for {
        tunnel: w1348 -> [w1379] mode=indexing
        tunnel: w1347 -> [w1378] mode=indexing
        tunnel: w1346 -> [w1377] mode=indexing
        shift-right: [w1376] -> w1349
        shift-left: w1350 -> [w1380]
        shift-right: [w1374] -> w1318
        shift-left: w1319 -> [w1375]
        n435 = Set Menu Item Info(7:w1379, 8:w1375, 9:w1377, 10:w1378, 11:w1380) -> (0:w1374:errorcluster, 3:w1376:refnum<k9>)  [unwired: 1 in, 1 out]
      }
      n436 = Insert Menu Items(5:w1354, 6:w1318, 7:w1362, 8:w1359, 9:w1349) -> (0:w1317:errorcluster, 3:w1371:refnum<k9>)  [unwired: 2 out]
      n437 = Insert Menu Items(5:w1353, 6:w1317, 7:w1361, 8:w1359, 9:w1371) -> (0:w1316:errorcluster, 3:w1370:refnum<k9>)  [unwired: 2 out]
      n438 = Insert Menu Items(5:w1352, 6:w1316, 7:w1363, 8:w1359, 9:w1370) -> (0:w1315:errorcluster, 3:w1369:refnum<k9>)  [unwired: 2 out]
      n439 = Insert Menu Items(5:w1351, 6:w1315, 7:w1364, 8:w1359, 9:w1369) -> (0:w1311:errorcluster, 3:w1313:refnum<k9>)  [unwired: 2 out]
      n440 = Not(x=w1307) -> (.not. x?=w1314:bool)
      n441 = Set Menu Item Info(7:w1308, 8:w1311, 9:w1314, 11:w1313) -> (0:w1310:errorcluster, 3:w1312:refnum<k9>)  [unwired: 1 in, 2 out]
      n442 = call "CRYGet Window Menu.vi"("Tags"=string[] ["DA_EXPORT_EXCEL", "DA_EXPORT_DOCUMENT"]) -> ("Tags_Out"=w1337:string[], "Names_Out"=w1338:string[])  [unwired: 8 in, 1 out]
      n443 = Insert Menu Items(5:w1332, 6:w1310, 7:w1337, 8:w1338, 9:w1312) -> (0:w1299:errorcluster, 1:w1301:string[], 3:w1300:refnum<k9>)  [unwired: 1 out]
      n444 = Index Array(array=w1301, index #1=0 ("index"), index #2=1 ("index")) -> (element #1=w1302:string, element #2=w1296:string)
      n445 = Set Menu Item Info(7:w1302, 8:w1299, 9:w1298, 11:w1300) -> (0:w1293:errorcluster, 3:w1295:refnum<k9>)  [unwired: 1 in, 2 out]
      n446 = Set Menu Item Info(7:w1296, 8:w1293, 9:w1291, 11:w1295) -> (0:w1292:errorcluster, 3:w1294:refnum<k9>)  [unwired: 1 in, 2 out]
    }
    frame "RESULT" {
      n447 = call "CRYGet Boolean Reference.vi"("Label Name"="Verdict", "VI Refnum"=w1418) -> ("Boolean Ref"=w1416:refnum<vi>)  [unwired: 7 in, 2 out]
      n448 = Delete Menu Items(9:w1457) -> (0:w1412:errorcluster, 3:w1458:refnum<k9>)  [unwired: 1 in, 2 out]
      n449 = property class="Bool"(reference=w1416) -> ("Visible"=w1413:bool)  [unwired: 1 in, 2 out]
      n450 = call "CRYGet Window Menu.vi"("Tags"=string[] ["DA_GRAPH", "DA_REMOVEONE", "DA_REMOVEALL", "APP_SEPARATOR", "DA_EXPORT", "APP_SEPARATOR", "DA_PROPERTY"]) -> ("Tags_Out"=w1422:string[], "Names_Out"=w1423:string[])  [unwired: 8 in, 1 out]
      n451 = Insert Menu Items(6:w1412, 7:w1422, 8:w1423, 9:w1458) -> (0:w1411:errorcluster, 1:w1453:string[], 3:w1396:refnum<k9>)  [unwired: 2 out]
      n452 = Select(t=FALSE, s=w1413, f=w1414) -> (s? t:f=w1388:bool)
      n453 = Index Array(array=w1453, index #1=0 ("index"), index #2=1 ("index"), index #3=2 ("index"), index #4=4 ("index")) -> (element #1=w1450:string, element #2=w1427:string, element #3=w1428:string, element #4=w1425:string)
      n454 = Set Menu Item Info(7:w1427, 8:w1411, 9:w1388, 11:w1396) -> (0:w1410:errorcluster, 3:w1426:refnum<k9>)  [unwired: 1 in, 2 out]
      n455 = Set Menu Item Info(7:w1428, 8:w1410, 9:w1388, 11:w1426) -> (0:w1394:errorcluster, 3:w1395:refnum<k9>)  [unwired: 1 in, 2 out]
      n456 = Insert Menu Items(5:w1450, 6:w1394, 7:w1445, 8:w1432, 9:w1395) -> (0:w1409:errorcluster, 1:w1433:string[], 3:w1435:refnum<k9>)  [unwired: 1 out]
      n457 = Index Array(array=w1433, index #1=0 ("index"), index #2=1 ("index"), index #3=2 ("index"), index #4=3 ("index"), index #5=4 ("index")) -> (element #1=w1439:string, element #2=w1438:string, element #3=w1437:string, element #4=w1436:string, element #5=w1400:string)
      n458 = for {
        tunnel: w1433 -> [w1464] mode=indexing
        tunnel: w1432 -> [w1463] mode=indexing
        tunnel: w1431 -> [w1462] mode=indexing
        shift-right: [w1461] -> w1434
        shift-left: w1435 -> [w1465]
        shift-right: [w1459] -> w1408
        shift-left: w1409 -> [w1460]
        n459 = Set Menu Item Info(7:w1464, 8:w1460, 9:w1462, 10:w1463, 11:w1465) -> (0:w1459:errorcluster, 3:w1461:refnum<k9>)  [unwired: 1 in, 1 out]
      }
      n460 = Insert Menu Items(5:w1439, 6:w1408, 7:w1447, 8:w1444, 9:w1434) -> (0:w1407:errorcluster, 3:w1456:refnum<k9>)  [unwired: 2 out]
      n461 = Insert Menu Items(5:w1438, 6:w1407, 7:w1446, 8:w1444, 9:w1456) -> (0:w1406:errorcluster, 3:w1455:refnum<k9>)  [unwired: 2 out]
      n462 = Insert Menu Items(5:w1437, 6:w1406, 7:w1448, 8:w1444, 9:w1455) -> (0:w1405:errorcluster, 3:w1454:refnum<k9>)  [unwired: 2 out]
      n463 = Insert Menu Items(5:w1436, 6:w1405, 7:w1449, 8:w1444, 9:w1454) -> (0:w1399:errorcluster, 3:w1403:refnum<k9>)  [unwired: 2 out]
      n464 = Not(x=w1397) -> (.not. x?=w1404:bool)
      n465 = Set Menu Item Info(7:w1400, 8:w1399, 9:w1404, 11:w1403) -> (0:w1398:errorcluster, 3:w1402:refnum<k9>)  [unwired: 1 in, 2 out]
      n466 = call "CRYGet Window Menu.vi"("Tags"=string[] ["DA_EXPORT_EXCEL", "DA_EXPORT_DOCUMENT"]) -> ("Tags_Out"=w1419:string[], "Names_Out"=w1420:string[])  [unwired: 8 in, 1 out]
      n467 = Insert Menu Items(5:w1425, 6:w1398, 7:w1419, 8:w1420, 9:w1402) -> (0:w1389:errorcluster, 1:w1391:string[], 3:w1390:refnum<k9>)  [unwired: 1 out]
      n468 = Index Array(array=w1391, index #1=0 ("index"), index #2=1 ("index")) -> (element #1=w1392:string, element #2=w1386:string)
      n469 = Set Menu Item Info(7:w1392, 8:w1389, 9:w1388, 11:w1390) -> (0:w1383:errorcluster, 3:w1385:refnum<k9>)  [unwired: 1 in, 2 out]
      n470 = Set Menu Item Info(7:w1386, 8:w1383, 9:w1381, 11:w1385) -> (0:w1382:errorcluster, 3:w1384:refnum<k9>)  [unwired: 1 in, 2 out]
    }
    frame "PICTURE" {
      n471 = Delete Menu Items(9:w1527) -> (0:w1495:errorcluster, 3:w1528:refnum<k9>)  [unwired: 1 in, 2 out]
      n472 = call "CRYGet Window Menu.vi"("Tags"=string[] ["DA_GRAPH", "APP_SEPARATOR", "DA_OPEN", "DA_DELETE", "APP_SEPARATOR", "DA_EXPORT", "APP_SEPARATOR", "DA_PROPERTY"]) -> ("Tags_Out"=w1496:string[], "Names_Out"=w1497:string[])  [unwired: 8 in, 1 out]
      n473 = Insert Menu Items(6:w1495, 7:w1496, 8:w1497, 9:w1528) -> (0:w1494:errorcluster, 1:w1523:string[], 3:w1501:refnum<k9>)  [unwired: 2 out]
      n474 = Index Array(array=w1523, index #1=0 ("index"), index #2=3 ("index"), index #3=5 ("index")) -> (element #1=w1521:string, element #2=w1500:string, element #3=w1474:string)
      n475 = Set Menu Item Info(7:w1500, 8:w1494, 9:w1499, 11:w1501) -> (0:w1493:errorcluster)  [unwired: 1 in, 3 out]
      n476 = Insert Menu Items(5:w1521, 6:w1493, 7:w1516, 8:w1504, 9:w1501) -> (0:w1492:errorcluster, 1:w1505:string[], 3:w1507:refnum<k9>)  [unwired: 1 out]
      n477 = Index Array(array=w1505, index #1=0 ("index"), index #2=1 ("index"), index #3=2 ("index"), index #4=3 ("index"), index #5=4 ("index")) -> (element #1=w1510:string, element #2=w1509:string, element #3=w1508:string, element #4=w1477:string, element #5=w1476:string)
      n478 = for {
        tunnel: w1505 -> [w1534] mode=indexing
        tunnel: w1504 -> [w1533] mode=indexing
        tunnel: w1503 -> [w1532] mode=indexing
        shift-right: [w1531] -> w1506
        shift-left: w1507 -> [w1535]
        shift-right: [w1529] -> w1491
        shift-left: w1492 -> [w1530]
        n479 = Set Menu Item Info(7:w1534, 8:w1530, 9:w1532, 10:w1533, 11:w1535) -> (0:w1529:errorcluster, 3:w1531:refnum<k9>)  [unwired: 1 in, 1 out]
      }
      n480 = Insert Menu Items(5:w1510, 6:w1491, 7:w1518, 8:w1515, 9:w1506) -> (0:w1490:errorcluster, 3:w1526:refnum<k9>)  [unwired: 2 out]
      n481 = Insert Menu Items(5:w1509, 6:w1490, 7:w1517, 8:w1515, 9:w1526) -> (0:w1489:errorcluster, 3:w1525:refnum<k9>)  [unwired: 2 out]
      n482 = Insert Menu Items(5:w1508, 6:w1489, 7:w1519, 8:w1515, 9:w1525) -> (0:w1488:errorcluster, 3:w1524:refnum<k9>)  [unwired: 2 out]
      n483 = Insert Menu Items(5:w1477, 6:w1488, 7:w1520, 8:w1515, 9:w1524) -> (0:w1486:errorcluster, 3:w1485:refnum<k9>)  [unwired: 2 out]
      n484 = Not(x=w1484) -> (.not. x?=w1487:bool)
      n485 = Set Menu Item Info(7:w1476, 8:w1486, 9:w1487, 11:w1485) -> (0:w1478:errorcluster, 3:w1479:refnum<k9>)  [unwired: 1 in, 2 out]
      n486 = call "CRYGet Window Menu.vi"("Tags"=string[] ["DA_EXPORT_DOCUMENT"]) -> ("Tags_Out"=w1480:string[], "Names_Out"=w1481:string[])  [unwired: 8 in, 1 out]
      n487 = Insert Menu Items(5:w1474, 6:w1478, 7:w1480, 8:w1481, 9:w1479) -> (0:w1468:errorcluster, 1:w1472:string[], 3:w1470:refnum<k9>)  [unwired: 1 out]
      n488 = Index Array(array=w1472, index=0) -> (element=w1471:string)
      n489 = Set Menu Item Info(7:w1471, 8:w1468, 9:w1466, 11:w1470) -> (0:w1467:errorcluster, 3:w1469:refnum<k9>)  [unwired: 1 in, 2 out]
    }
    frame "TEXT" {
      n490 = Open Application Reference() -> (0:w1565:errorcluster, 3:w1564:refnum<vi>)  [unwired: 4 in]
      n491 = Delete Menu Items(9:w1600) -> (0:w1557:errorcluster, 3:w1601:refnum<k9>)  [unwired: 1 in, 2 out]
      n492 = invoke class="App" method="Clipboard.Read"(reference=w1564, error in=w1565) -> (error out=w1563:errorcluster, "Read Clipbrd"=w1539:string)  [unwired: 1 in, 1 out]
      n493 = call "CRYGet Window Menu.vi"("Tags"=string[] ["DA_GRAPH", "APP_SEPARATOR", "DA_CUT", "DA_COPY", "DA_PASTE", "DA_CLEAR", "APP_SEPARATOR", "DA_PROPERTY"]) -> ("Tags_Out"=w1558:string[], "Names_Out"=w1559:string[])  [unwired: 8 in, 1 out]
      n494 = Insert Menu Items(6:w1557, 7:w1558, 8:w1559, 9:w1601) -> (0:w1556:errorcluster, 1:w1561:string[], 3:w1571:refnum<k9>)  [unwired: 2 out]
      n495 = Empty String/Path?(string/path=w1539) -> (empty?=w1540:bool)
      n496 = case shown="No Error" w1563 {
        frame No Error {
        }
        frame Error {
        }
      }
      n497 = Not(x=w1540) -> (.not. x?=w1538:bool)
      n498 = Index Array(array=w1561, index #1=0 ("index"), index #2=2 ("index"), index #3=3 ("index"), index #4=4 ("index"), index #5=5 ("index")) -> (element #1=w1595:string, element #2=w1576:string, element #3=w1570:string, element #4=w1569:string, element #5=w1568:string)
      n499 = Set Menu Item Info(7:w1576, 8:w1556, 9:w1566, 11:w1571) -> (0:w1555:errorcluster)  [unwired: 1 in, 3 out]
      n500 = Set Menu Item Info(7:w1570, 8:w1555, 9:w1566, 11:w1571) -> (0:w1554:errorcluster)  [unwired: 1 in, 3 out]
      n501 = Set Menu Item Info(7:w1569, 8:w1554, 9:w1538, 11:w1571) -> (0:w1553:errorcluster)  [unwired: 1 in, 3 out]
      n502 = Set Menu Item Info(7:w1568, 8:w1553, 9:w1567, 11:w1571) -> (0:w1552:errorcluster)  [unwired: 2 in, 2 out]
      n503 = Insert Menu Items(5:w1595, 6:w1552, 7:w1590, 8:w1578, 9:w1571) -> (0:w1551:errorcluster, 1:w1579:string[], 3:w1562:refnum<k9>)  [unwired: 1 out]
      n504 = Index Array(array=w1579, index #1=0 ("index"), index #2=1 ("index"), index #3=2 ("index"), index #4=3 ("index"), index #5=4 ("index")) -> (element #1=w1584:string, element #2=w1583:string, element #3=w1582:string, element #4=w1581:string, element #5=w1541:string)
      n505 = for {
        tunnel: w1579 -> [w1607] mode=indexing
        tunnel: w1578 -> [w1606] mode=indexing
        tunnel: w1577 -> [w1605] mode=indexing
        shift-right: [w1604] -> w1580
        shift-left: w1562 -> [w1608]
        shift-right: [w1602] -> w1550
        shift-left: w1551 -> [w1603]
        n506 = Set Menu Item Info(7:w1607, 8:w1603, 9:w1605, 10:w1606, 11:w1608) -> (0:w1602:errorcluster, 3:w1604:refnum<k9>)  [unwired: 1 in, 1 out]
      }
      n507 = Insert Menu Items(5:w1584, 6:w1550, 7:w1592, 8:w1589, 9:w1580) -> (0:w1549:errorcluster, 3:w1599:refnum<k9>)  [unwired: 2 out]
      n508 = Insert Menu Items(5:w1583, 6:w1549, 7:w1591, 8:w1589, 9:w1599) -> (0:w1548:errorcluster, 3:w1598:refnum<k9>)  [unwired: 2 out]
      n509 = Insert Menu Items(5:w1582, 6:w1548, 7:w1593, 8:w1589, 9:w1598) -> (0:w1547:errorcluster, 3:w1597:refnum<k9>)  [unwired: 2 out]
      n510 = Insert Menu Items(5:w1581, 6:w1547, 7:w1594, 8:w1589, 9:w1597) -> (0:w1544:errorcluster, 3:w1545:refnum<k9>)  [unwired: 2 out]
      n511 = Not(x=w1543) -> (.not. x?=w1546:bool)
      n512 = Set Menu Item Info(7:w1541, 8:w1544, 9:w1546, 11:w1545) -> (0:w1536:errorcluster, 3:w1537:refnum<k9>)  [unwired: 1 in, 2 out]
    }
    frame "LEGEND" {
      n513 = Delete Menu Items(9:w1619) -> (0:w1614:errorcluster, 3:w1618:refnum<k9>)  [unwired: 1 in, 2 out]
      n514 = case shown="Default" w1609 {
        tunnel: [w1648 w1653] -> w1620
        tunnel: w1618 -> [w1648 w1652]
        tunnel: w1616 -> [_ w1651]
        tunnel: w1614 -> [w1647 w1650]
        tunnel: [w1647 w1649] -> w1613
        frame "INTENSITY" {
        }
        frame Default {
          n515 = case shown="True" w1651 {
            tunnel: w1652 -> [w1655 w1661]
            tunnel: [w1655 w1662] -> w1653
            tunnel: w1650 -> [w1654 w1657]
            tunnel: [w1654 w1656] -> w1649
            frame False {
            }
            frame True {
              n516 = call "CRYGet Window Menu.vi"("Tags"=string[] ["DA_LEG_REMOVE"]) -> ("Tags_Out"=w1658:string[], "Names_Out"=w1659:string[])  [unwired: 8 in, 1 out]
              n517 = Insert Menu Items(6:w1657, 7:w1658, 8:w1659, 9:w1661) -> (0:w1656:errorcluster, 3:w1662:refnum<k9>)  [unwired: 3 out]
            }
          }
        }
      }
      n518 = case shown="True" w1615 {
        tunnel: w1620 -> [w1664 w1672]
        tunnel: [w1664 w1671] -> w1617
        tunnel: w1609 -> [_ w1670]
        tunnel: w1613 -> [w1663 w1666]
        tunnel: [w1663 w1665] -> w1612
        frame False {
        }
        frame True {
          n519 = case shown="Default" w1670 {
            tunnel: [string[] ["DA_LEG_REMOVEALL", "APP_SEPARATOR", "DA_LEG_SHOWALL", "DA_LEG_INVERT", "APP_SEPARATOR"] string[] ["DA_LEG_REMOVE"]] -> w1669
            frame Default {
            }
            frame "INTENSITY" {
            }
          }
          n520 = call "CRYGet Window Menu.vi"("Tags"=w1669) -> ("Tags_Out"=w1667:string[], "Names_Out"=w1668:string[])  [unwired: 8 in, 1 out]
          n521 = Insert Menu Items(6:w1666, 7:w1667, 8:w1668, 9:w1672) -> (0:w1665:errorcluster, 3:w1671:refnum<k9>)  [unwired: 3 out]
        }
      }
      n522 = case shown="Default" w1609 {
        tunnel: w1617 -> [w1640 w1646]
        tunnel: w1612 -> [w1639 w1645]
        tunnel: [w1623 w1641] -> w1611
        tunnel: w1610 -> [w1621 _]
        frame Default {
          n523 = call "CRYGet Window Menu.vi"("Tags"=string[] ["DA_LEG_SHOW", "APP_SEPARATOR", "DA_LEG_HIDE_1"] ("item tags")) -> ("Tags_Out"=w1637:string[], "Names_Out"=w1638:string[])  [unwired: 8 in, 1 out]
          n524 = Insert Menu Items(6:w1639, 7:w1637, 8:w1638, 9:w1640) -> (0:w1624:errorcluster, 1:w1635:string[], 3:w1622:refnum<k9>)  [unwired: 2 out]
          n525 = Index Array(array=w1635, index=0) -> (element=w1625:string)
          n526 = Select(t="DA_LEG_VSCROLL_HIDE", s=w1621, f="DA_LEG_VSCROLL_VIEW") -> (s? t:f=w1630:string)
          n527 = Build Array(w1630) -> (w1633:string[])
          n528 = call "CRYGet Window Menu.vi"("Tags"=w1633) -> ("Names_Out"=w1632:string[])  [unwired: 8 in, 2 out]
          n529 = Index Array(array=w1632) -> (element=w1629:string)  [unwired: 1 in]
          n530 = Insert Menu Items(5:w1625, 6:w1624, 7:w1630, 8:w1629, 9:w1622) -> (0:w1626:errorcluster, 3:w1631:refnum<k9>)  [unwired: 2 out]
          n531 = Set Menu Item Info(6:w1621, 7:w1630, 8:w1626, 10:w1629, 11:w1631) -> (0:w1623:errorcluster)  [unwired: 1 in, 2 out]
        }
        frame "INTENSITY" {
          n532 = call "CRYGet Window Menu.vi"("Tags"=string[] ["DA_LEG_HIDE_1"] ("item tags")) -> ("Tags_Out"=w1643:string[], "Names_Out"=w1644:string[])  [unwired: 8 in, 1 out]
          n533 = Insert Menu Items(6:w1645, 7:w1643, 8:w1644, 9:w1646) -> (0:w1641:errorcluster)  [unwired: 4 out]
        }
      }
    }
    frame "FREQUENCY" {
      n534 = Delete Menu Items(9:w1701) -> (0:w1696:errorcluster, 3:w1700:refnum<k9>)  [unwired: 1 in, 2 out]
      n535 = case shown="True" w1699 {
        tunnel: w1700 -> [w1704 w1710]
        tunnel: [w1704 w1711] -> w1702
        tunnel: w1696 -> [w1703 w1706]
        tunnel: [w1703 w1705] -> w1695
        frame False {
        }
        frame True {
          n536 = call "CRYGet Window Menu.vi"("Tags"=string[] ["DA_FREQ_REMOVE"]) -> ("Tags_Out"=w1707:string[], "Names_Out"=w1708:string[])  [unwired: 8 in, 1 out]
          n537 = Insert Menu Items(6:w1706, 7:w1707, 8:w1708, 9:w1710) -> (0:w1705:errorcluster, 3:w1711:refnum<k9>)  [unwired: 3 out]
        }
      }
      n538 = case shown="True" w1698 {
        tunnel: w1702 -> [w1713 w1720]
        tunnel: [w1713 w1719] -> w1677
        tunnel: w1697 -> [_ _]
        tunnel: w1695 -> [w1712 w1715]
        tunnel: [w1712 w1714] -> w1678
        frame False {
        }
        frame True {
          n539 = call "CRYGet Window Menu.vi"("Tags"=string[] ["DA_FREQ_REMOVEALL", "APP_SEPARATOR", "DA_FREQ_SHOWALL", "DA_FREQ_INVERT", "APP_SEPARATOR"]) -> ("Tags_Out"=w1716:string[], "Names_Out"=w1717:string[])  [unwired: 8 in, 1 out]
          n540 = Insert Menu Items(6:w1715, 7:w1716, 8:w1717, 9:w1720) -> (0:w1714:errorcluster, 3:w1719:refnum<k9>)  [unwired: 3 out]
        }
      }
      n541 = call "CRYGet Window Menu.vi"("Tags"=string[] ["DA_FREQ_SHOW", "APP_SEPARATOR", "DA_FREQ_HIDE_1"] ("item tags")) -> ("Tags_Out"=w1693:string[], "Names_Out"=w1694:string[])  [unwired: 8 in, 1 out]
      n542 = Insert Menu Items(6:w1678, 7:w1693, 8:w1694, 9:w1677) -> (0:w1680:errorcluster, 1:w1691:string[], 3:w1679:refnum<k9>)  [unwired: 2 out]
      n543 = Index Array(array=w1691, index=0) -> (element=w1681:string)
      n544 = Select(t="DA_FREQ_VSCROLL_HIDE", s=w1675, f="DA_FREQ_VSCROLL_VIEW") -> (s? t:f=w1686:string)
      n545 = Build Array(w1686) -> (w1689:string[])
      n546 = call "CRYGet Window Menu.vi"("Tags"=w1689) -> ("Names_Out"=w1688:string[])  [unwired: 8 in, 2 out]
      n547 = Index Array(array=w1688) -> (element=w1685:string)  [unwired: 1 in]
      n548 = Insert Menu Items(5:w1681, 6:w1680, 7:w1686, 8:w1685, 9:w1679) -> (0:w1682:errorcluster, 3:w1687:refnum<k9>)  [unwired: 2 out]
      n549 = Set Menu Item Info(6:w1675, 7:w1686, 8:w1682, 10:w1685, 11:w1687) -> (0:w1676:errorcluster)  [unwired: 1 in, 2 out]
    }
    frame "CURSOR" {
      n550 = Delete Menu Items(9:w1737) -> (0:w1724:errorcluster, 3:w1736:refnum<k9>)  [unwired: 1 in, 2 out]
      n551 = case shown="\"INTENSITY\"" w1725 {
        selector: w1725 -> [w1745 _]
        tunnel: w1736 -> [w1780 w1810]
        tunnel: [w1755 w1803] -> w1733
        tunnel: [w1754 w1804] -> w1731
        tunnel: w1730 -> [w1753 _]
        tunnel: w1729 -> [w1752 _]
        tunnel: w1724 -> [w1744 w1802]
        tunnel: [w1738 w1801] -> w1723
        frame "OCTAVE", "WAVE", "XY", Default {
          n552 = case shown="\"OCTAVE\", \"XY\"" w1745 {
            tunnel: w1752 -> [w1789 w1796]
            tunnel: [w1785 w1792] -> w1767
            tunnel: [w1784 w1791] -> w1758
            frame "WAVE", Default {
              n553 = Variant To Data(type=refnum<vi> refnum ("WaveGraph Ref"), Variant=w1789) -> (data=w1788:refnum<vi>)  [unwired: 1 in, 1 out]
              n554 = property class="WFGraph"(reference=w1788, "Active Cursor"=u32 0, "Active Cursor"=u32 1) -> ("Cursor.Cursor Plot"=w1785:i32, "Cursor.Cursor Plot"=w1784:i32)  [unwired: 1 in, 2 out]
            }
            frame "OCTAVE", "XY" {
              n555 = Variant To Data(type=refnum<vi> refnum ("XY Graph"), Variant=w1796) -> (data=w1793:refnum<vi>)  [unwired: 1 in, 1 out]
              n556 = property class="XYGraph"(reference=w1793, "Active Cursor"=u32 0, "Active Cursor"=u32 1) -> ("Cursor.Cursor Plot"=w1792:i32, "Cursor.Cursor Plot"=w1791:i32)  [unwired: 1 in, 2 out]
            }
          }
          n557 = call "CRYGet Window Menu.vi"("Tags"=string[] ["DA_CUR_LINKTO", "DA_CUR_GOTO", "DA_BRING_CENTER", "APP_SEPARATOR", "DA_CUR_PRO"]) -> ("Tags_Out"=w1749:string[], "Names_Out"=w1750:string[])  [unwired: 8 in, 1 out]
          n558 = Insert Menu Items(6:w1744, 7:w1749, 8:w1750, 9:w1780) -> (0:w1743:errorcluster, 1:w1778:string[], 3:w1775:refnum<k9>)  [unwired: 1 in, 1 out]
          n559 = Index Array(array=w1778, index #1=0 ("index"), index #2=1 ("index")) -> (element #1=w1776:string, element #2=w1754:string)
          n560 = call "CRYGet Window Menu.vi"("Tags"=string[] ["DA_CUR_LINK_CUR#0", "DA_CUR_LINK_CUR#1"]) -> ("Tags_Out"=w1746:string[], "Names_Out"=w1747:string[])  [unwired: 8 in, 1 out]
          n561 = Insert Menu Items(5:w1776, 6:w1743, 7:w1746, 8:w1747, 9:w1775) -> (0:w1742:errorcluster, 1:w1772:string[], 3:w1774:refnum<k9>)  [unwired: 1 in]
          n562 = Index Array(array=w1772, index #1=0 ("index"), index #2=1 ("index")) -> (element #1=w1770:string, element #2=w1769:string)
          n563 = for {
            tunnel: w1753 -> [w1799] mode=indexing
            tunnel: [w1800] -> w1766 mode=indexing
            tunnel: "LINKTO#0_" -> [w1798]
            n564 = Concatenate Strings(w1798, w1799) -> (w1800:string)
          }
          n565 = Index Array(array=w1766, index=w1767) -> (element=w1765:string)
          n566 = Insert Menu Items(5:w1770, 6:w1742, 7:w1766, 8:w1753, 9:w1774) -> (0:w1741:errorcluster, 3:w1768:refnum<k9>)  [unwired: 1 in, 1 out]
          n567 = Set Menu Item Info(6:TRUE ("checked"), 7:w1765, 8:w1741, 9:TRUE ("enabled"), 11:w1768) -> (0:w1740:errorcluster)  [unwired: 3 out]
          n568 = for {
            tunnel: w1753 -> [w1782] mode=indexing
            tunnel: [w1783] -> w1759 mode=indexing
            tunnel: "LINKTO#1_" -> [w1781]
            n569 = Concatenate Strings(w1781, w1782) -> (w1783:string)
          }
          n570 = Insert Menu Items(5:w1769, 6:w1740, 7:w1759, 8:w1753, 9:w1768) -> (0:w1739:errorcluster, 3:w1755:refnum<k9>)  [unwired: 1 in, 1 out]
          n571 = Index Array(array=w1759, index=w1758) -> (element=w1757:string)
          n572 = Set Menu Item Info(6:TRUE ("checked"), 7:w1757, 8:w1739, 9:TRUE ("enabled"), 11:w1755) -> (0:w1738:errorcluster)  [unwired: 3 out]
        }
        frame "INTENSITY" {
          n573 = call "CRYGet Window Menu.vi"("Tags"=string[] ["DA_CUR_GOTO", "APP_SEPARATOR", "DA_CUR_PRO"]) -> ("Tags_Out"=w1805:string[], "Names_Out"=w1806:string[])  [unwired: 8 in, 1 out]
          n574 = Insert Menu Items(6:w1802, 7:w1805, 8:w1806, 9:w1810) -> (0:w1801:errorcluster, 1:w1808:string[], 3:w1803:refnum<k9>)  [unwired: 1 in, 1 out]
          n575 = Index Array(array=w1808, index=0) -> (element=w1804:string)
        }
      }
      n576 = call "CRYGet Window Menu.vi"("Tags"=string[] ["DA_CUR_GOTO_CUR#0", "DA_CUR_GOTO_CUR#1"]) -> ("Tags_Out"=w1726:string[], "Names_Out"=w1727:string[])  [unwired: 8 in, 1 out]
      n577 = Insert Menu Items(5:w1731, 6:w1723, 7:w1726, 8:w1727, 9:w1733) -> (0:w1722:errorcluster, 3:w1732:refnum<k9>)  [unwired: 1 in, 1 out]
      n578 = case shown="False" w1734 {
        tunnel: w1732 -> [w1812 w1823]
        tunnel: [w1812 w1822] -> w1735
        tunnel: w1722 -> [w1811 w1815]
        tunnel: [w1811 w1813] -> w1721
        frame False {
        }
        frame True {
          n579 = call "CRYGet Window Menu.vi"("Tags"=string[] ["APP_SEPARATOR"] ("item tags")) -> ("Tags_Out"=w1819:string[], "Names_Out"=w1820:string[])  [unwired: 8 in, 1 out]
          n580 = Insert Menu Items(6:w1815, 7:w1819, 8:w1820, 9:w1823) -> (0:w1814:errorcluster, 3:w1824:refnum<k9>)  [unwired: 3 out]
          n581 = call "CRYGet Window Menu.vi"("Tags"=string[] ["DA_CUR_HIDE_1"]) -> ("Tags_Out"=w1816:string[], "Names_Out"=w1817:string[])  [unwired: 8 in, 1 out]
          n582 = Insert Menu Items(6:w1814, 7:w1816, 8:w1817, 9:w1824) -> (0:w1813:errorcluster, 3:w1822:refnum<k9>)  [unwired: 3 out]
        }
      }
    }
    frame "PREVIEW" {
      n583 = Delete Menu Items(9:w1832) -> (0:w1826:errorcluster, 3:w1831:refnum<k9>)  [unwired: 1 in, 2 out]
      n584 = call "CRYGet Window Menu.vi"("Tags"=string[] ["DA_PRE_SHOWALL", "DA_PRE_LOCATION", "APP_SEPARATOR", "DA_PRE_HIDE_1"]) -> ("Tags_Out"=w1827:string[], "Names_Out"=w1828:string[])  [unwired: 8 in, 1 out]
      n585 = Insert Menu Items(6:w1826, 7:w1827, 8:w1828, 9:w1831) -> (0:w1825:errorcluster, 3:w1830:refnum<k9>)  [unwired: 1 in, 2 out]
    }
    frame Default {
      # "INTENSITY"
      n586 = Delete Menu Items(9:w1835) -> (0:w1833:errorcluster, 3:w1834:refnum<k9>)  [unwired: 1 in, 2 out]
    }
  }
  "Runtime Menu Ref Out" <- w53
  n587 = call "CRYCurve Library Error Message.vi"("sAction"="Menu", "error IO"=w2) -> ()  [unwired: 10 in]
